vi "MegaAwesome_10_10_12b_JW.vi"() -> ()   [LabVIEW 2011]
uses:
  data/MegaAwesome_States.ctl
  <vilib>/Utility/inputDevices.llb/keyboardAcquire.vi
  <vilib>/Utility/file.llb/Read From Spreadsheet File (string).vi
  <vilib>/Utility/file.llb/Write To Spreadsheet File (string).vi
panel:
  out "Save Next?":bool
  out "Image Center X":i32
  in  "Disable Flag":bool
  out "Index":string
  in  "Slider Min":dbl=5.0
  in  "Slider Max":dbl=5.0
  out "Opj X Axis":string
  out "X Axis Display Type":string
  in  "Index-Sat":dbl=5.0
  in  "Index-Lin":dbl=5.0
  in  "IndexLog-Lin":dbl=5.0
  in  "IndexLog-Sat":dbl=5.0 caption="Num Pts"
  out "Lin Id-Log Used":dbl[](array[numeric])
  out "Lin-Vg Array-Log Used":dbl[](array[numeric])
  in  "New: Comments":string
  out "Save Array":string[][](array[string])
  out "Folder Index":i32 caption="Length"
  out "Sat Id-Used":dbl[](array[numeric])
  out "Sat Vg Array-Used":dbl[](array[numeric])
  out "Vg Array-Log-Used":dbl[](array[numeric])
  out "Sat Id-Log-Used":dbl[](array[numeric])
  out "Lin Id-Used":dbl[](array[numeric])
  out "Lin-Vg Array-Used":dbl[](array[numeric])
  out "Lin Vd":dbl
  out "Recorded Prop":T1
  out "Current State":T2
  in  "Main Tab Control":T3(tab)
  in  "Transfer File":path
  out "Transfer Folder":path
  in  "Transport\nFolder":path caption="Transport Folder"
  out "Transport\nFile":path caption="Transport File"
  in  "Image Folder":path
  out "Image File":path
  out "Fabrication Prop":T4
  out "Distances":i32[](array[numeric])
  in  "Zoom":i32(slide)=-3 scale=-5.0..5.0
  in  "Magnification":i32(ring) items=["5x", "10x", "20x", "50x", "80x"]
  in  "Undo Button":bool
  in  "Remove Button":bool
  in  "Transfer Plots":T5(tab)=enum."Saturation"
  in  "Lin-Trans Slider":dbl(slide) step=1.0 scale=-40.0..40.0 scale format="%#_1p"
  out "Sqrt-Lin":cluster{dbl[], dbl[]}[](graph)
  in  "Sat-Trans Slider":dbl(slide) step=1.0 scale=-40.0..40.0 scale format="%#_1p"
  out "Sqrt-Sat":cluster{dbl[], dbl[]}[](graph)
  out "Raw- Lin":cluster{dbl[], dbl[]}[](graph)
  out "Raw- Sat":cluster{dbl[], dbl[]}[](graph)
  in  "Log Plots":enum32{"Linear", "Saturation", "Transport"}(tab)=enum."Saturation"
  in  "Lin-Log Slider":dbl(slide) step=1.0 scale=-40.0..40.0 scale format="%#_1p"
  out "Lin-Log":cluster{dbl[], dbl[]}[](graph)
  in  "Sat-Log Slider":dbl(slide) step=1.0 scale=-40.0..40.0 scale format="%#_1p"
  out "Sat-Log":cluster{dbl[], dbl[]}[](graph)
  out "Transport":cluster{ext[], ext[]}[](graph)
  out "Transport Name:":string
  in  "Manual Controls":T6
  in  "File Controls":T7
  out "Date Recorded":string="Date Recorded" caption="Measured"
  out "Data Name:":string
  out "Image Name":string
  out "Date Created":string caption="Fabricated"
  in  "Comments:":string
  out "Rec: Length":dbl caption="Length" format="%#_3g"
  out "Rec: Width":dbl caption="Width" format="%#_4g"
  out "Rec: Dielectric (d)":dbl caption="Dielectric (d)" format="%#_3g"
  in  "New: Dielectric":dbl
  in  "New: Length":dbl
  in  "New: Width":dbl
  out "Rec: Temp":dbl caption="Sample Temp" format="%.1f"
  in  "New: Temp":dbl format="%.1f"
  out "Image Out":T8(plugin-control)
  in  "Num Pts":dbl=5.0
  in  "Num Pts Log":dbl=5.0 caption="Num Pts"
  out "Recorded Values Cluster":T9
  out "Calculated Values Cluster":T9 caption="Recorded Values Cluster"
  out "Re-Calculated Values Cluster":T9 caption="Recorded Values Cluster"
  in  "Independant Variable:":string(combo)="Length (um):"
  out "Image Preview":T8(plugin-control)
  out "Total Width":i32
  in  "Index Array":i32(ring) caption="Index" items=["4C", "4C", "4C", "4C", "4C", "4C", "4C", "4C", "4C", "4C", "4C", "4C", "4C", "4C", "4C", "4C", "4C", "4C", "4C", "4C", "4C", "4C", "4C", "4C", "4C", "4C", "4C", "4C", "4C", "4C", "4C", "4C", "4C", "4C", "4C", "4C", "4C", "4C", "4C"]
  in  "Room Temp":dbl=294.0 caption="Room Temp (K)"
  out "No Image\n File":path=path "\\\\acad1\\physics/Jurchescu-group/JW-PD/Mega Awesome/Image Not Found.png" caption="No Image File"
  out "Origin Project File":path=path "\\\\acad1\\physics/Jurchescu-group/JW-PD/Group Library/Origin Project Files/DeviceData_8_10_12a_JW.opj"
  out "No Transport\n File":path=path "\\\\acad1\\physics/Jurchescu-group/JW-PD/Mega Awesome/No Transport File.txt" caption="No Transport File"
  in  "Transport Style Controls":T10={"Transport Line Size"=1, "Transport Line Color"=16772608} {"Transport Line Size" items=["Extra Small", "Small", "Medium", "Large", "Extra Large"]}
  out "Application Directory":path
  # "1)  Select the Transfer File that you would like to analyze:"
  # "Transfer Location"
  # "2) What else would you like to view during your analysis?"
  # "Transport Location"
  # "Image Location"
  # "Recorded"
  # "Calculated"
  # "Re-Calculated"
  # "Manual"
  # "um"
  # "Slider\nDoesn't\nWork"
  # "V"
  # "V"
  # "Slider\nDoesn't\nWork"
  # "V"
  # "Default File Choices"
  # "Default Analysis Values"
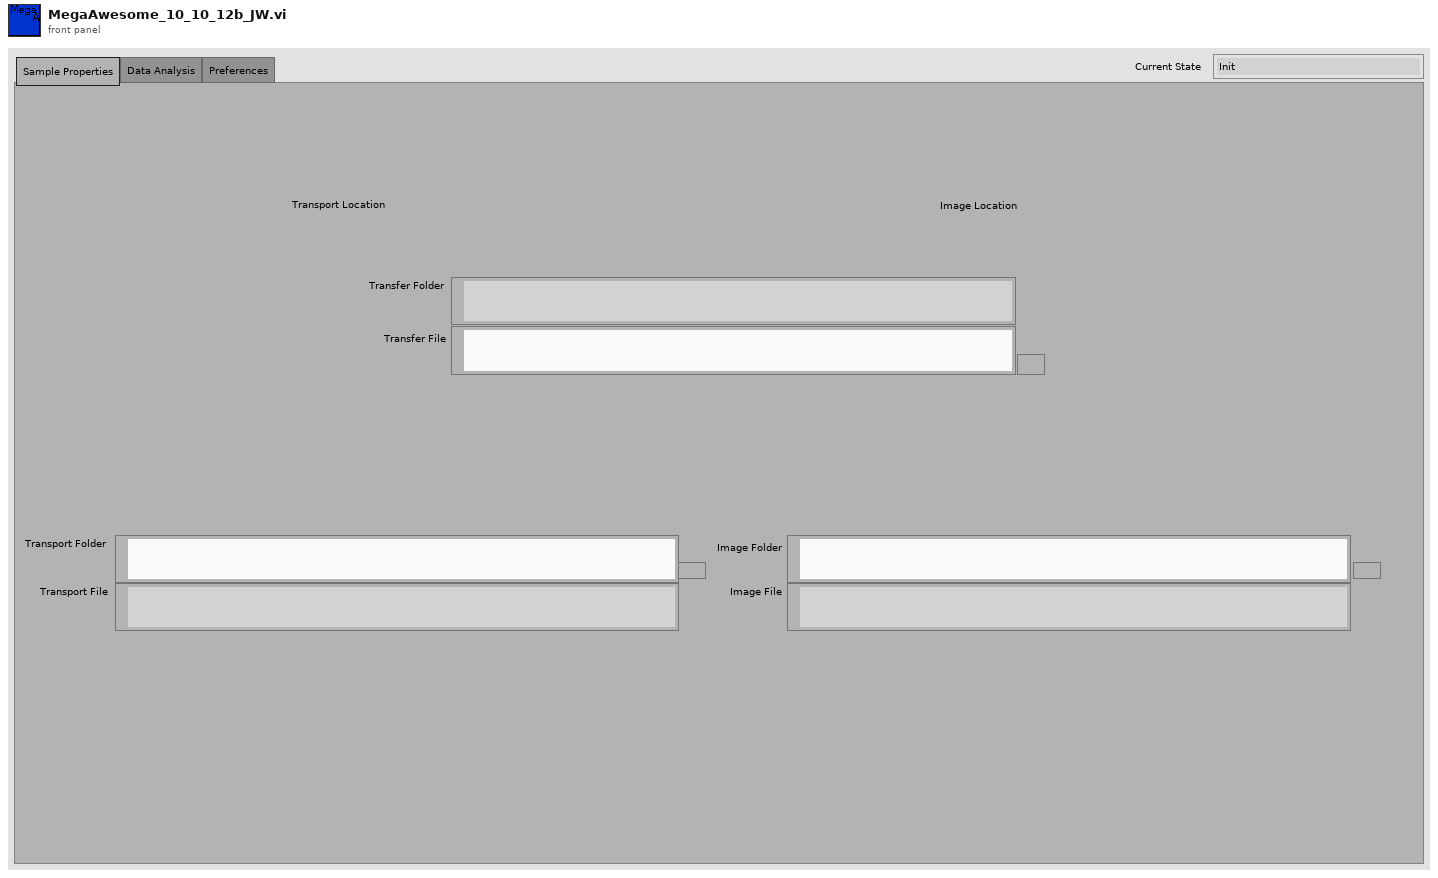
[diagram p1: front panel]
types:
  T1 = cluster{"Date Recorded":string, "Index":string, "Length":dbl, "Width":dbl, "Sample Temp":dbl}
  T2 = typedef "MegaAwesome_States.ctl" = enum16{"Init", "File Missing", "No Event", "Read Data", "Calculated Values", "Re-Calculated Values", "Next File", "Previous File", "Discard File", "Save", "Save Lines", "Export", "Exit"}
  T3 = enum32{"Sample Properties", "Data Analysis", "Preferences"}
  T4 = cluster{"Date Created":string, "Material":string, "Solvent":string, "Concentration":dbl, "Method":string, "Dielectric (nm)":dbl, "Treatment":string, "Comments":string}
  T5 = enum32{"Linear", "Saturation", "Raw-Linear", "Raw-Saturation"}
  T6 = cluster{"Manual-Temp":bool, "Manual-Width":bool, "Manuel-Length":bool, "Manuel-Dielectric":bool, "Manual Comments":bool}
  T7 = cluster{"Previous File":bool, "Discard ":bool, "Save Lines":bool, "Close":bool, "Next File ":bool, "Save":bool, "Save Next":bool, "Export":bool}
  T8 = typedef "IMAQ Image.ctl" = refnum<image>
  T9 = cluster{"Mobility-Sat":dbl, "Moblitity-Lin":dbl, "On/Off":dbl, "Off Current":dbl, "Vt-Sat":dbl, "STS":dbl, "Trap Density-VT":dbl, "Trap Density-STS":dbl}
  T10 = cluster{"Transport Line Size":u16, "Transport Line Color":u32}
  T11 = typedef "LVBoundsTypeDef.ctl" = cluster{"Width":u32, "Height":u32}
  T12 = enum16{"0", "1", "2", "3", "4", "5", "6", "7", "8", "9", "A", "B", "C", "D", "E", "F", "G", "H", "I", "J", "K", "L", "M", "N", "O", "P", "Q", "R", "S", "T", "U", "V", "W", "X", "Y", "Z", "F1", "F2", "F3", "F4", "F5", "F6", "F7", "F8", "F9", "F10", "F11", "F12", "F13", "F14", "F15", "ADD", "BACK", "BACKSLASH", "CAPITAL", "COMMA", "DECIMAL", "DELETE", "DIVIDE", "DOWN", "END", "EQUALS", "ESCAPE", "GRAVE (`)", "HOME", "INSERT", "LBRACKET", "LCONTROL", "LEFT", "L ALT", "LSHIFT", "LWIN", "MINUS", "MULTIPLY", "NEXT", "NUMLOCK", "NUMPAD_0", "NUMPAD_1", "NUMPAD_2", "NUMPAD_3", "NUMPAD_4", "NUMPAD_5", "NUMPAD_6", "NUMPAD_7", "NUMPAD_8", "NUMPAD_9", "PAUSE", "PERIOD", "PRIOR (PG UP)", "RBRACKET", "RCONTROL", "RETURN", "RIGHT", "R ALT", "RSHIFT", "RWIN", "SCROLL", "SEMICOLON", "SLASH", "SPACE", "SUBTRACT", "TAB", "UP", "ENTER (num pad)", "' (quote)"}[]
  T13 = enum16{"0", "1", "2", "3", "4", "5", "6", "7", "8", "9", "A", "B", "C", "D", "E", "F", "G", "H", "I", "J", "K", "L", "M", "N", "O", "P", "Q", "R", "S", "T", "U", "V", "W", "X", "Y", "Z", "F1", "F2", "F3", "F4", "F5", "F6", "F7", "F8", "F9", "F10", "F11", "F12", "F13", "F14", "F15", "ADD", "BACK", "BACKSLASH", "CAPITAL", "COMMA", "DECIMAL", "DELETE", "DIVIDE", "DOWN", "END", "EQUALS", "ESCAPE", "GRAVE (`)", "HOME", "INSERT", "LBRACKET", "LCONTROL", "LEFT", "L ALT", "LSHIFT", "LWIN", "MINUS", "MULTIPLY", "NEXT", "NUMLOCK", "NUMPAD_0", "NUMPAD_1", "NUMPAD_2", "NUMPAD_3", "NUMPAD_4", "NUMPAD_5", "NUMPAD_6", "NUMPAD_7", "NUMPAD_8", "NUMPAD_9", "PAUSE", "PERIOD", "PRIOR (PG UP)", "RBRACKET", "RCONTROL", "RETURN", "RIGHT", "R ALT", "RSHIFT", "RWIN", "SCROLL", "SEMICOLON", "SLASH", "SPACE", "SUBTRACT", "TAB", "UP", "ENTER (num pad)", "' (quote)"}
  T14 = typedef "ROI Descriptor" = cluster{"Global Rectangle":i32[], "Contours":cluster{"ID":enum32{"External", "Internal"}, "Type":u32, "Coordinates":i32[]}[]}
  T15 = cluster{string, dbl, bool, bool, bool, bool, bool, bool, i32}
  T16 = cluster{i32, cluster{string, dbl, bool, bool, bool, bool, bool, bool, i32}, i32, i32}
  T17 = cluster{"Global Rectangle":i32[], "Contours":cluster{"Contour Type":u32, "ROI Type":u32, "Points":i32[]}[]}
  T18 = cluster{"Contour Type":u32, "ROI Type":u32, "Points":i32[]}[]
  T19 = cluster{"[0]":cluster{dbl[], dbl[]}, "[1]":cluster{dbl[], dbl[]}, "[2]":cluster{dbl[], dbl[]}, "[3]":cluster{dbl[], dbl[]}, "[4]":cluster{dbl[], dbl[]}, "[5]":cluster{dbl[], dbl[]}, "[6]":cluster{dbl[], dbl[]}, "[7]":cluster{dbl[], dbl[]}, "[8]":cluster{dbl[], dbl[]}}
  T20 = cluster{i32[], cluster{"Contour Type":u32, "ROI Type":u32, "Points":i32[]}[]}
  T21 = cluster{"Contour Type":u32, "ROI Type":u32, "Points":i32[]}
  T22 = cluster{"Points[0]":i32, "Points[1]":i32, "Points[2]":i32, "Points[3]":i32, "Points[4]":i32, "Points[5]":i32, "Points[6]":i32, "Points[7]":i32, "Points[8]":i32}
  T23 = cluster{"Sat Vg Used":dbl[], "Sat Sqrt(Id) Used ":dbl[], "Lin Vg Used":dbl[], "Lin Sqrt(Id) Used":dbl[], "Index-Lin":dbl, "Index-Sat":dbl}
  T24 = cluster{"Raw Sat":cluster{dbl[], dbl[]}[], "Sqrt Sat":cluster{dbl[], dbl[]}[], "Log Sat":cluster{dbl[], dbl[]}[], "Raw Lin":cluster{dbl[], dbl[]}[], "Sqrt Lin":cluster{dbl[], dbl[]}[], "Log Lin":cluster{dbl[], dbl[]}[]}
  T25 = cluster{"Mobility-Sat":dbl, "Vt-Sat":dbl, "Mobility-Lin":dbl, "Vt-Lin":dbl, "Off I-Sat":dbl, "On/Off I-Sat":dbl}
  T26 = cluster{"Sat Vg Used":dbl[], "Sat Log(Id) Used":dbl[], "Lin Vg Used":dbl[], "Lin Log(Id) Used":dbl[], "STS Index-Sat":dbl, "STS Index-Lin":dbl}
  T27 = cluster{"Independant  Variable Indicator":string, "Parameter String Indicator":string}
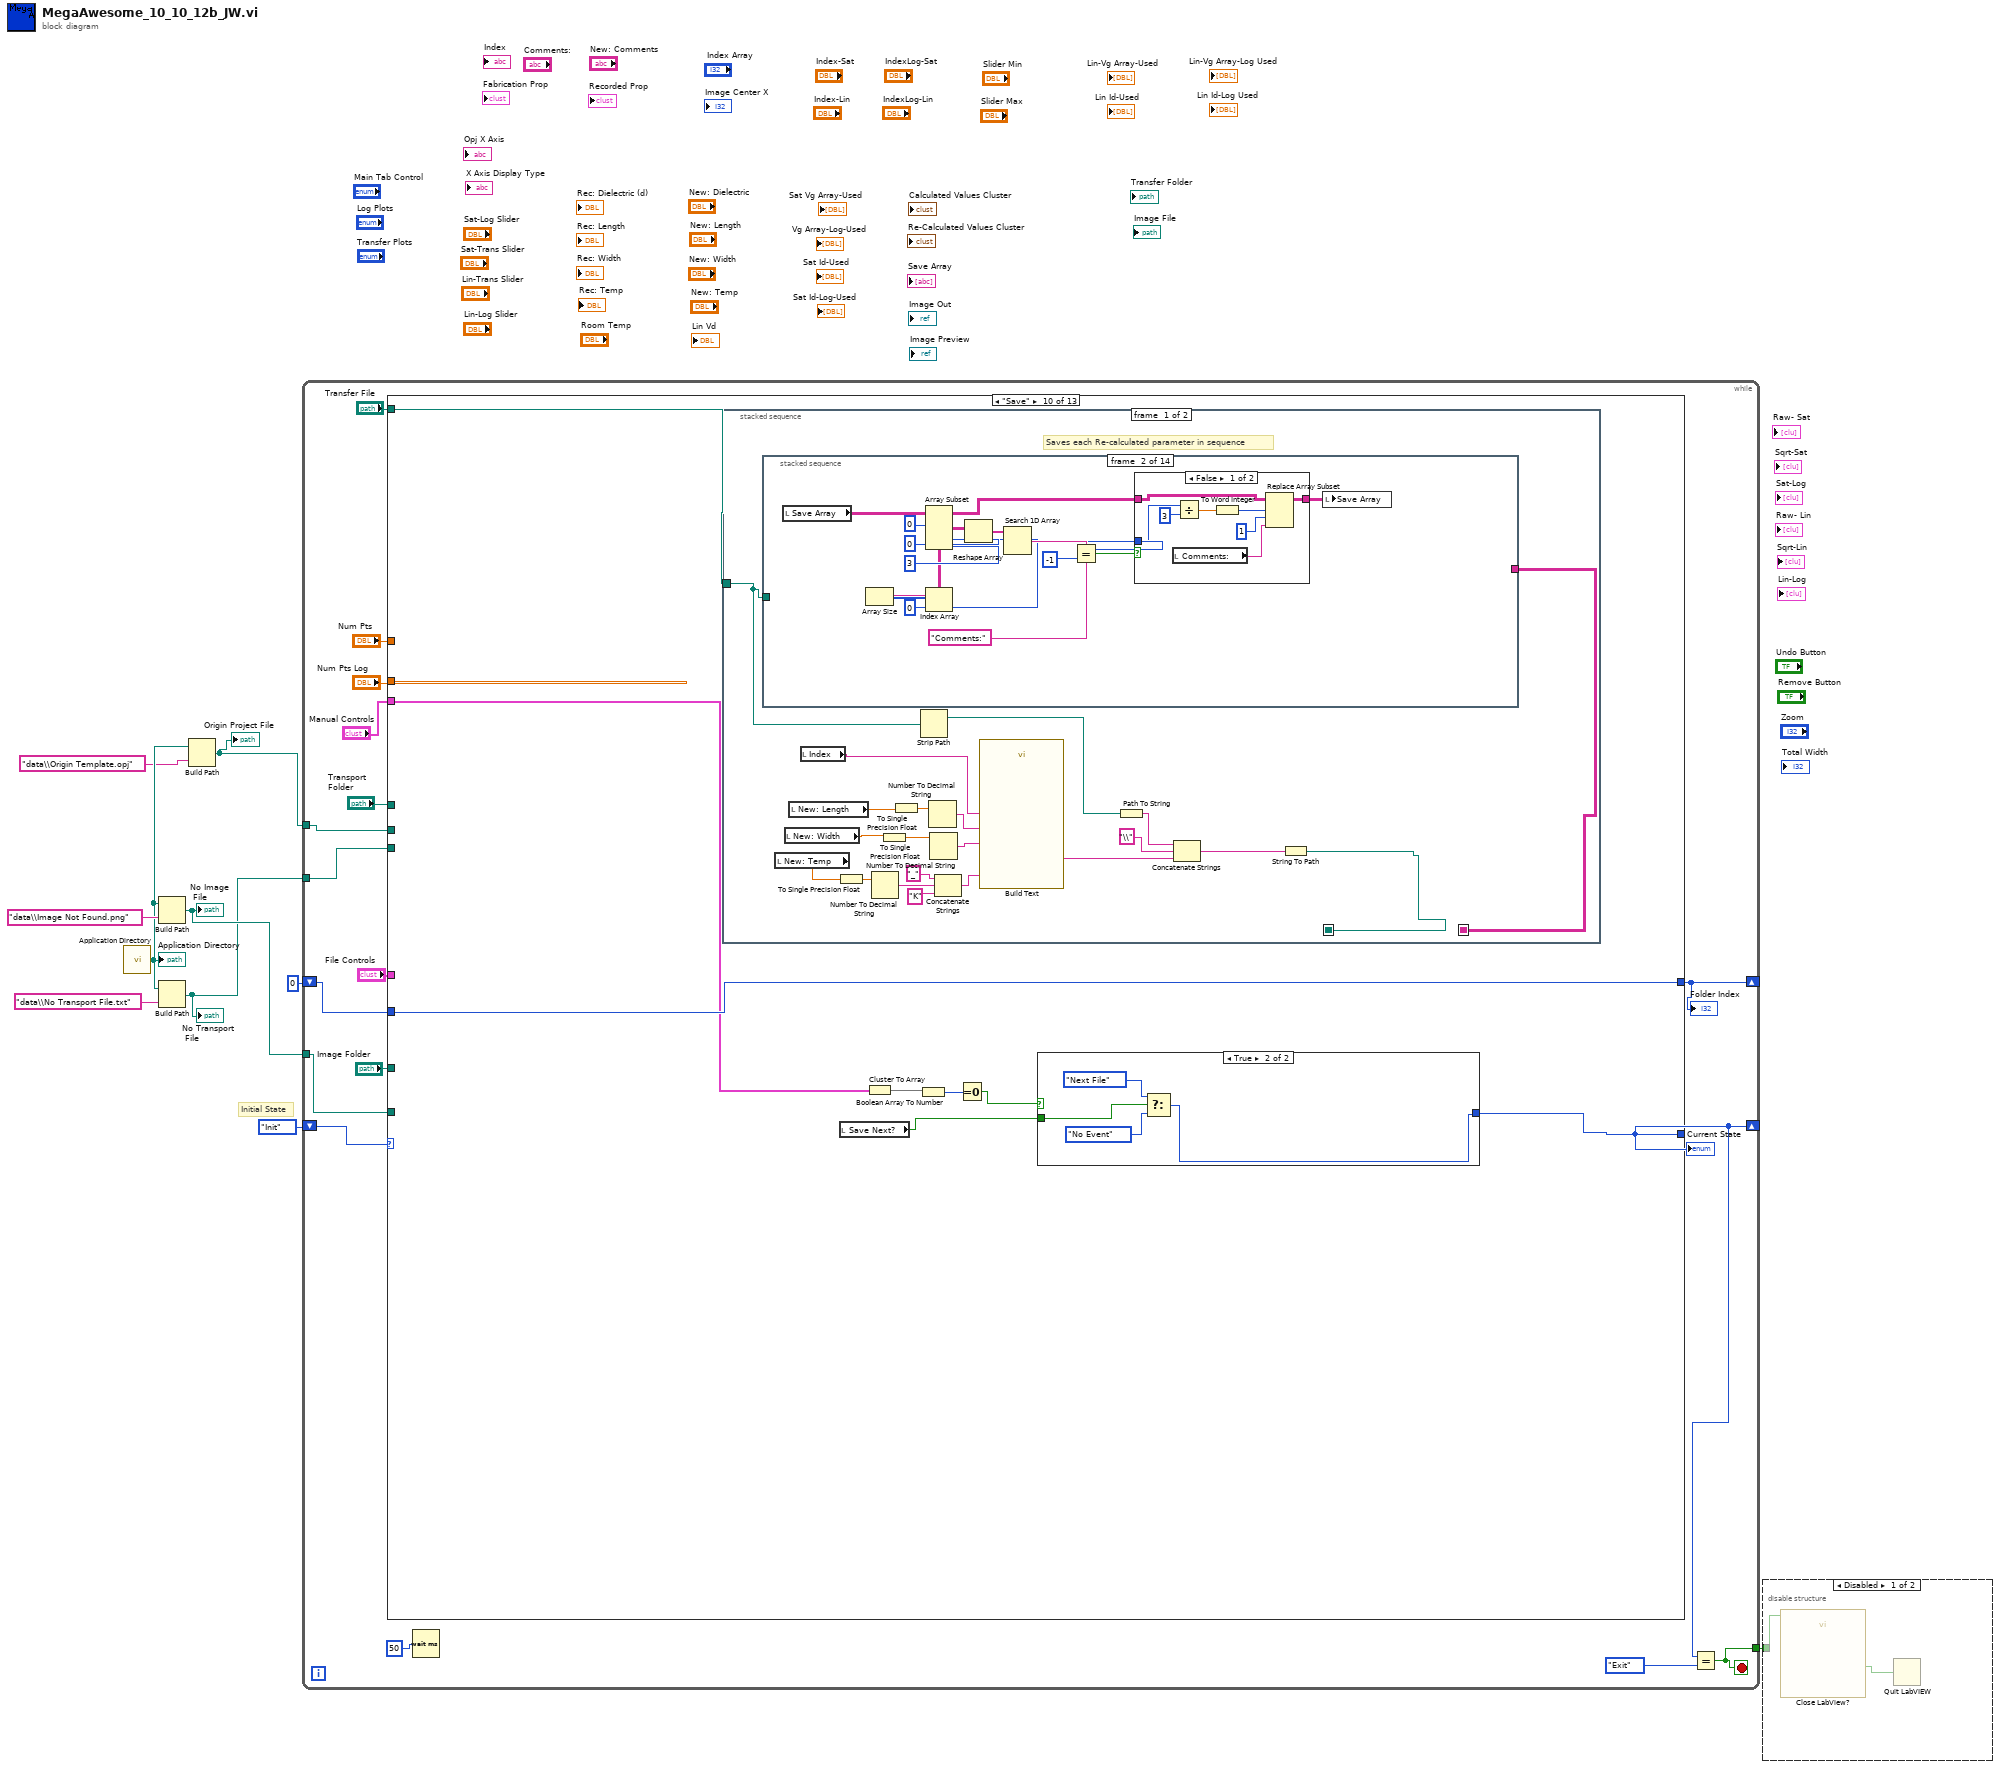
[diagram p0: block diagram]
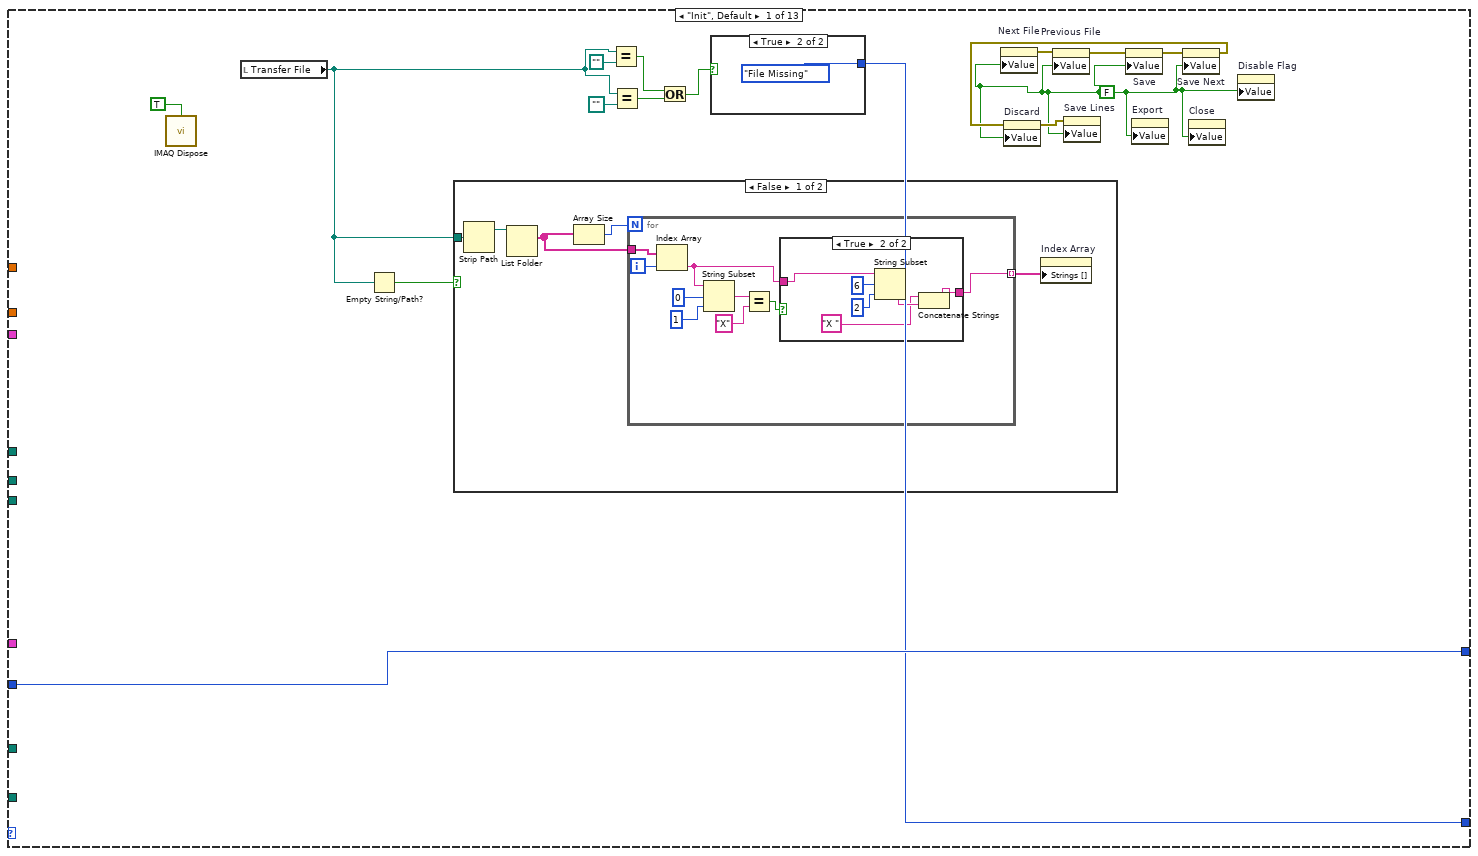
[diagram p3: hidden frame]
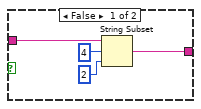
[diagram p4: hidden frame]
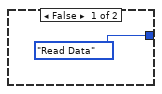
[diagram p6: hidden frame]
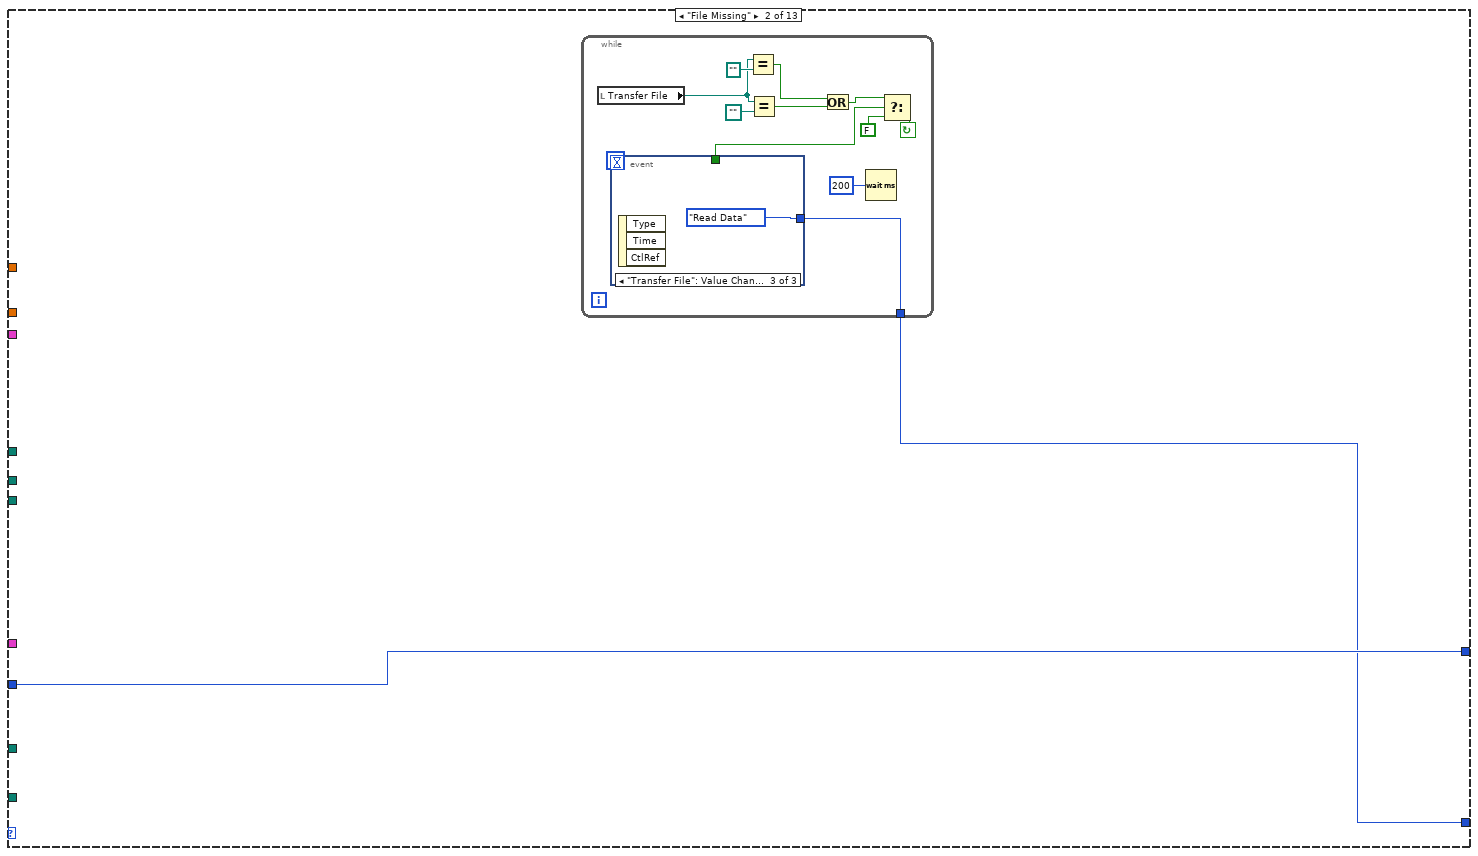
[diagram p7: hidden frame]
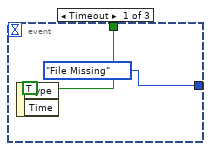
[diagram p8: hidden frame]
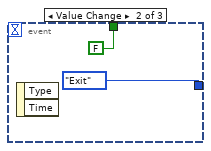
[diagram p9: hidden frame]
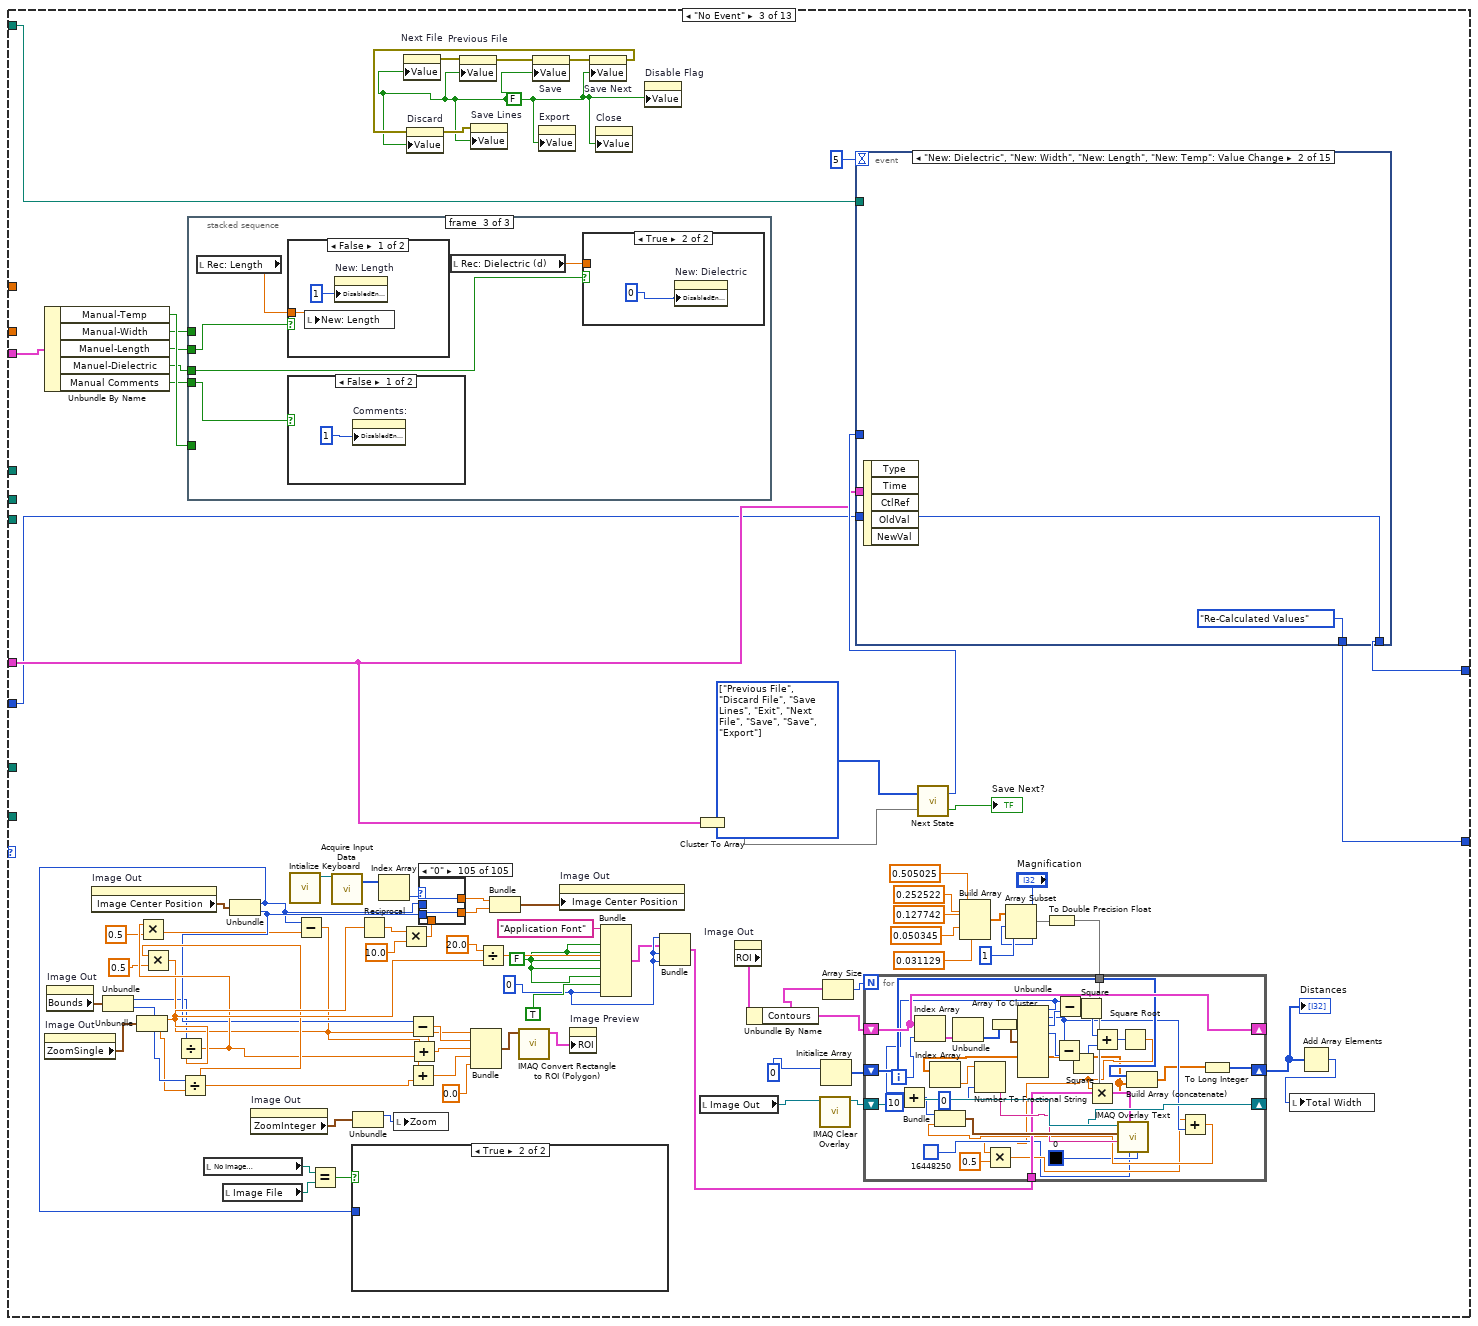
[diagram p10: hidden frame]
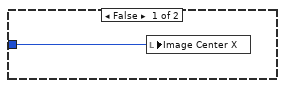
[diagram p11: hidden frame]
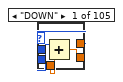
[diagram p12: hidden frame]
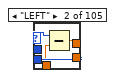
[diagram p13: hidden frame]
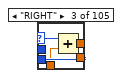
[diagram p14: hidden frame]
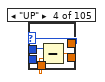
[diagram p15: hidden frame]
diagram:
  # "Initial State"
  n1 = call <vilib>:"Application Directory.vi"() -> ("Application Directory"=w3:path)
  "Application Directory" <- w3
  n2 = Build Path(base path=w3, name or relative path="data\\Image Not Found.png") -> (appended path=w6:path)
  "No Image\n File" <- w6
  n3 = Build Path(base path=w3, name or relative path="data\\No Transport File.txt") -> (appended path=w5:path)
  "No Transport\n File" <- w5
  n4 = Build Path(base path=w3, name or relative path="data\\Origin Template.opj") -> (appended path=w4:path)
  "Origin Project File" <- w4
  n5 = while {
    shift-right: [w11] -> _
    shift-left: MegaAwesome_States."Init" -> [w13]
    shift-right: [w21] -> _
    shift-left: 0 -> [w22]
    tunnel: w6 -> [w18]
    tunnel: w5 -> [w16]
    tunnel: w4 -> [w15]
    tunnel: [w14] -> w1
    stop <- w14 stop-if-true
    n6 = case shown="\"Save\"" w13 {
      tunnel: [w28 w70 w164 MegaAwesome_States."Calculated Values" MegaAwesome_States."Re-Calculated Values" MegaAwesome_States."No Event" MegaAwesome_States."Read Data" MegaAwesome_States."Read Data" MegaAwesome_States."Init" w816 MegaAwesome_States."Exit" MegaAwesome_States."No Event" MegaAwesome_States."No Event"] -> w11
      tunnel: "Transfer File" -> [_ _ w156 w615 w663 _ w764 w775 w802 w821 _ _ _]
      tunnel: "Num Pts" -> [_ _ _ _ w698 _ _ _ _ _ _ _ _]
      tunnel: "Num Pts Log" -> [_ _ _ _ w697 _ _ _ _ _ _ _ _]
      tunnel: "Image Folder" -> [_ _ _ _ w694 _ _ _ _ _ _ w1351 _]
      tunnel: w18 -> [_ _ _ _ w693 _ _ _ _ _ _ _ _]
      tunnel: [w38 w71 w157 w620 w692 w724 w750 w773 w798 w822 w1337 w1361 w1367] -> w21
      tunnel: w22 -> [w38 w71 w89 w618 w692 w724 w751 w774 _ w822 w1337 w1361 w1367]
      tunnel: "Manual Controls" -> [_ _ w166 _ _ _ _ _ _ w820 _ _ _]
      tunnel: "File Controls" -> [_ _ w154 _ _ _ _ _ _ _ _ _ _]
      tunnel: "Transport\nFolder" -> [_ _ _ _ w659 _ _ _ _ _ _ _ _]
      tunnel: w16 -> [_ _ _ _ w658 _ _ _ _ _ _ _ _]
      tunnel: w15 -> [_ _ _ _ _ _ _ _ _ _ _ _ w1366]
      frame "Init", Default {
        w29 = FALSE
        n7 = call "IMAQ Dispose"("All Images? (No)"=TRUE) -> ()  [unwired: 5 in, 1 out]
        n8 = local read "Transfer File"() -> (w36:path)
        n9 = Empty String/Path?(string/path=w36) -> (empty?=w37:bool)
        n10 = case shown="False" w37 {
          tunnel: w36 -> [w45 _]
          frame False {
            n11 = Strip Path(path=w45) -> (stripped path=w47:path)  [unwired: 1 out]
            n12 = List Folder(path=w47) -> (filenames=w46:string[])  [unwired: 3 in, 3 out]
            n13 = Array Size(array=w46) -> (size(s)=w48:i32)
            n14 = for {
              N: w48 -> [_]
              tunnel: w46 -> [w57]
              tunnel: [w55] -> w44 mode=indexing
              i -> [w56]
              n15 = Index Array(array=w57, index=w56) -> (element=w54:string)
              n16 = String Subset(string=w54, offset (0)=0, length (rest)=1) -> (substring=w51:string)
              n17 = Equal?(x=w51, y="X") -> (x = y?=w50:bool)
              n18 = case shown="True" w50 {
                tunnel: w54 -> [w61 w65]
                tunnel: [w58 w64] -> w55
                frame False {
                  n19 = String Subset(string=w61, offset (0)=4, length (rest)=2) -> (substring=w58:string)
                }
                frame True {
                  n20 = String Subset(string=w65, offset (0)=6, length (rest)=2) -> (substring=w63:string)
                  n21 = Concatenate Strings("X ", w63) -> (w64:string)
                }
              }
            }
            n22 = property on="Index Array" class="Ring (strict)"("Strings []"=w44) -> ()  [unwired: 2 in, 2 out]
          }
          frame True {
          }
        }
        n23 = Equal?(x=w36, y=path "") -> (x = y?=w41:bool)
        n24 = Equal?(x=w36, y=path "") -> (x = y?=w40:bool)
        n25 = Or(x=w41, y=w40) -> (x .or. y?=w43:bool)
        n26 = case shown="True" w43 {
          tunnel: [MegaAwesome_States."Read Data" MegaAwesome_States."File Missing"] -> w28
          frame False {
          }
          frame True {
          }
        }
        n27 = property on="Next File" class="Bool (strict)"("Value"=w29) -> (error out=w34:errorcluster)  [unwired: 2 in, 1 out]
        n28 = property on="Previous File" class="Bool (strict)"(error in=w34, "Value"=w29) -> (error out=w33:errorcluster)  [unwired: 1 in, 1 out]
        n29 = property on="Save" class="Bool (strict)"(error in=w33, "Value"=w29) -> (error out=w32:errorcluster)  [unwired: 1 in, 1 out]
        n30 = property on="Export" class="Bool (strict)"("Value"=w29) -> ()  [unwired: 2 in, 2 out]
        n31 = property on="Save Next" class="Bool (strict)"(error in=w32, "Value"=w29) -> (error out=w31:errorcluster)  [unwired: 1 in, 1 out]
        n32 = property on="Discard" class="Bool (strict)"(error in=w31, "Value"=w29) -> (error out=w30:errorcluster)  [unwired: 1 in, 1 out]
        n33 = property on="Save Lines" class="Bool (strict)"(error in=w30, "Value"=w29) -> ()  [unwired: 1 in, 2 out]
        n34 = property on="Close" class="Bool (strict)"("Value"=w29) -> ()  [unwired: 2 in, 2 out]
        n35 = property on="Disable Flag" class="Bool (strict)"("Value"=w29) -> ()  [unwired: 2 in, 2 out]
      }
      frame "File Missing" {
        n36 = while {
          tunnel: [w78] -> w70
          stop <- w74 continue-if-true
          n37 = local read "Transfer File"() -> (w79:path)
          n38 = event shown="[2] \"Transfer File\": Value Change" {
            selector: _ -> [_ _ _]
            dyn-events: _ -> [_ _ _]
            timeout: 10 -> [_ _ _]
            tunnel: [MegaAwesome_States."File Missing" MegaAwesome_States."Exit" MegaAwesome_States."Read Data"] -> w78
            tunnel: [TRUE FALSE _] -> w77
            event Timeout {
              n39 = event-data() -> ()  [unwired: 1 in, 2 out]
            }
            event "File Controls.Close": Value Change {
              n40 = event-data() -> ()  [unwired: 1 in, 2 out]
            }
            event "Transfer File": Value Change {
              n41 = event-data() -> ()  [unwired: 1 in, 3 out]
            }
          }
          n42 = Equal?(x=w79, y=path "") -> (x = y?=w81:bool)
          n43 = Equal?(x=w79, y=path "") -> (x = y?=w82:bool)
          n44 = Or(x=w81, y=w82) -> (x .or. y?=w76:bool)
          n45 = Wait (ms)(milliseconds to wait=u32 200) -> ()  [unwired: 1 out]
          n46 = Select(t=w76, s=w77, f=FALSE) -> (s? t:f=w74:bool)
        }
      }
      frame "No Event" {
        w145 = FALSE
        w147 = 0
        w155 = FALSE
        w173 = T2[] [enum."Previous File", enum."Discard File", enum."Save Lines", enum."Exit", enum."Next File", enum."Save", enum."Save", enum."Export"] items=["Init", "File Missing", "No Event", "Read Data", "Calculated Values", "Re-Calculated Values", "Next File", "Previous File", "Discard File", "Save", "Save Lines", "Export", "Exit"]
        n47 = Unbundle By Name(w166) -> ("Manual-Temp"=w171:bool, "Manual-Width"=w170:bool, "Manuel-Length"=w169:bool, "Manuel-Dielectric"=w168:bool, "Manual Comments"=w167:bool)
        n48 = property on="Image Out" class="ImageControl"() -> ("ZoomSingle"=w131:cluster{"X":sgl, "Y":sgl})  [unwired: 2 in, 2 out]
        n49 = property on="Image Out" class="ImageControl"() -> ("Bounds"=w130:T11)  [unwired: 2 in, 2 out]
        n50 = property on="Image Out" class="ImageControl"() -> ("Image Center Position"=w124:cluster{"X":u32, "Y":u32})  [unwired: 2 in, 2 out]
        n51 = Unbundle(w130) -> ("Width"=w133:u32, "Height"=w134:u32)
        n52 = Unbundle(w131) -> ("X"=w151:sgl, "Y"=w132:sgl)
        n53 = Divide(x=w133, y=w151) -> (x/y=w142:sgl)
        n54 = Multiply(x=w142, y=0.5) -> (x*y=w137:dbl)
        n55 = Divide(x=w134, y=w132) -> (x/y=w143:sgl)
        n56 = Multiply(x=w143, y=0.5) -> (x*y=w138:dbl)
        n57 = stacked-sequence {
          tunnel: w171 -> [w573 _ _]
          tunnel: w170 -> [_ w587 _]
          tunnel: w169 -> [_ _ w600]
          tunnel: w168 -> [_ _ w598]
          tunnel: w167 -> [_ _ w597]
          frame #0 {
            n58 = local read "Rec: Temp"() -> (w572:dbl)
            n59 = case shown="False" w573 {
              tunnel: w572 -> [w578 _]
              frame False {
                n60 = local read "Rec: Temp"() -> (w576:dbl)
                n61 = property on="New: Temp" class="DigNum (strict)"("DisabledEnum"=1) -> ()  [unwired: 2 in, 2 out]
                n62 = Equal To 0?(x=w576) -> (x = 0?=w577:bool)
                n63 = local write "New: Temp"(w578) -> ()
                n64 = case shown="True" w577 {
                  tunnel: [w579 w580] -> w574
                  tunnel: w576 -> [w579 _]
                  frame False {
                  }
                  frame True {
                    n65 = local read "Room Temp"() -> (w580:dbl)
                  }
                }
                n66 = local write "Rec: Temp"(w574) -> ()
                n67 = local write "New: Temp"(w574) -> ()
              }
              frame True {
                n68 = property on="New: Temp" class="DigNum (strict)"("DisabledEnum"=0) -> ()  [unwired: 2 in, 2 out]
              }
            }
          }
          frame #1 {
            n69 = local read "New: Width"() -> (w588:dbl)
            n70 = local read "Total Width"() -> (w584:i32)
            n71 = case shown="True" w587 {
              frame False {
                n72 = property on="New: Width" class="DigNum (strict)"("DisabledEnum"=1) -> ()  [unwired: 2 in, 2 out]
              }
              frame True {
                n73 = property on="New: Width" class="DigNum (strict)"("DisabledEnum"=0) -> ()  [unwired: 2 in, 2 out]
              }
            }
            n74 = Not(x=w587) -> (.not. x?=w582:bool)
            n75 = Not Equal?(x=w584, y=w588) -> (x != y?=w583:bool)
            n76 = Equal To 0?(x=w584) -> (x = 0?=w586:bool)
            n77 = And(x=w582, y=w586) -> (x .and. y?=w585:bool)
            n78 = case shown="False" w585 {
              tunnel: w584 -> [w592 _]
              tunnel: w583 -> [w591 _]
              tunnel: w582 -> [w590 _]
              frame False {
                n79 = And(x=w590, y=w591) -> (x .and. y?=w589:bool)
                n80 = case shown="True" w589 {
                  tunnel: w592 -> [_ w593]
                  frame False {
                  }
                  frame True {
                    n81 = property on="New: Width" class="DigNum (strict)"("Val(Sgnl)"=w593) -> ()  [unwired: 2 in, 2 out]
                  }
                }
              }
              frame True {
                n82 = local read "Rec: Width"() -> (w594:dbl)
                n83 = local write "New: Width"(w594) -> ()
              }
            }
          }
          frame #2 {
            n84 = local read "Rec: Length"() -> (w601:dbl)
            n85 = case shown="False" w600 {
              tunnel: w601 -> [w608 _]
              frame False {
                n86 = local write "New: Length"(w608) -> ()
                n87 = property on="New: Length" class="DigNum (strict)"("DisabledEnum"=u8 1) -> ()  [unwired: 2 in, 2 out]
              }
              frame True {
                n88 = property on="New: Length" class="DigNum (strict)"("DisabledEnum"=0) -> ()  [unwired: 2 in, 2 out]
              }
            }
            n89 = case shown="False" w597 {
              frame False {
                n90 = property on="Comments:" class="Str"("DisabledEnum"=1) -> ()  [unwired: 2 in, 2 out]
              }
              frame True {
                n91 = property on="Comments:" class="Str"("DisabledEnum"=0) -> ()  [unwired: 2 in, 2 out]
              }
            }
            n92 = local read "Rec: Dielectric (d)"() -> (w599:dbl)
            n93 = case shown="True" w598 {
              tunnel: w599 -> [w605 _]
              frame False {
                n94 = local write "New: Dielectric"(w605) -> ()
                n95 = property on="New: Dielectric" class="DigNum (strict)"("DisabledEnum"=1) -> ()  [unwired: 2 in, 2 out]
              }
              frame True {
                n96 = property on="New: Dielectric" class="DigNum (strict)"("DisabledEnum"=0) -> ()  [unwired: 2 in, 2 out]
              }
            }
          }
        }
        n97 = local read "No Image\n File"() -> (w95:path)
        n98 = local read "Image File"() -> (w94:path)
        n99 = Unbundle(w124) -> ("X"=w96:u32, "Y"=w141:u32)
        n100 = property on="Image Out" class="ImageControl"() -> ("ZoomInteger"=w99:cluster{"X":i32, "Y":i32})  [unwired: 2 in, 2 out]
        n101 = call <vilib>:"Intialize Keyboard.vi"() -> ("device ID"=w121:refnum<k1>)  [unwired: 10 in, 1 out]
        n102 = Subtract(x=w96, y=w137) -> (x-y=w139:dbl)
        n103 = Equal?(x=w95, y=w94) -> (x = y?=w93:bool)
        n104 = call-poly <vilib>:"Acquire Input Data.vi"("device ID"=w121) -> ("keys pressed"=w122:T12)  [unwired: 16 in, 2 out]
        n105 = case shown="True" w93 {
          tunnel: w96 -> [w174 _]
          frame False {
            n106 = local write "Image Center X"(w174) -> ()
          }
          frame True {
          }
        }
        n107 = Unbundle(w99) -> ("X"=w98:i32)  [unwired: 1 out]
        n108 = Reciprocal(x=w151) -> (1/x=w152:sgl)
        n109 = Index Array(array=w122) -> (element=w118:T13)  [unwired: 1 in]
        n110 = local write "Zoom"(w98) -> ()
        n111 = Multiply(x=w152, y=sgl 10.0) -> (x*y=w150:sgl)
        n112 = property on="Next File" class="Bool (strict)"("Value"=w155) -> (error out=w162:errorcluster)  [unwired: 2 in, 1 out]
        n113 = Subtract(x=w141, y=w138) -> (x-y=w140:dbl)
        n114 = Add(x=w140, y=w143) -> (x+y=w126:dbl)
        n115 = Add(x=w139, y=w142) -> (x+y=w125:dbl)
        n116 = case shown="\"0\"" w118 {
          tunnel: w96 -> [w210 w216 w220 w222 w226 w228 w230 w232 w234 w236 w238 w240 w242 w244 w246 w248 w250 w252 w254 w256 w258 w260 w262 w264 w266 w268 w270 w272 w274 w276 w278 w280 w282 w284 w286 w288 w290 w292 w294 w296 w298 w300 w302 w304 w306 w308 w310 w312 w314 w316 w318 w320 w322 w324 w326 w328 w330 w332 w334 w336 w338 w340 w342 w344 w346 w348 w350 w352 w354 w356 w358 w360 w362 w364 w366 w368 w370 w372 w374 w376 w378 w380 w382 w384 w386 w388 w390 w392 w394 w396 w398 w400 w402 w404 w406 w408 w410 w412 w414 w416 w418 w420 w422 w424 w426]
          tunnel: [w210 w215 w219 w222 w226 w228 w230 w232 w234 w236 w238 w240 w242 w244 w246 w248 w250 w252 w254 w256 w258 w260 w262 w264 w266 w268 w270 w272 w274 w276 w278 w280 w282 w284 w286 w288 w290 w292 w294 w296 w298 w300 w302 w304 w306 w308 w310 w312 w314 w316 w318 w320 w322 w324 w326 w328 w330 w332 w334 w336 w338 w340 w342 w344 w346 w348 w350 w352 w354 w356 w358 w360 w362 w364 w366 w368 w370 w372 w374 w376 w378 w380 w382 w384 w386 w388 w390 w392 w394 w396 w398 w400 w402 w404 w406 w408 w410 w412 w414 w416 w418 w420 w422 w424 w426] -> w119
          tunnel: w141 -> [w212 w214 w218 w224 w225 w227 w229 w231 w233 w235 w237 w239 w241 w243 w245 w247 w249 w251 w253 w255 w257 w259 w261 w263 w265 w267 w269 w271 w273 w275 w277 w279 w281 w283 w285 w287 w289 w291 w293 w295 w297 w299 w301 w303 w305 w307 w309 w311 w313 w315 w317 w319 w321 w323 w325 w327 w329 w331 w333 w335 w337 w339 w341 w343 w345 w347 w349 w351 w353 w355 w357 w359 w361 w363 w365 w367 w369 w371 w373 w375 w377 w379 w381 w383 w385 w387 w389 w391 w393 w395 w397 w399 w401 w403 w405 w407 w409 w411 w413 w415 w417 w419 w421 w423 w425]
          tunnel: [w211 w214 w218 w223 w225 w227 w229 w231 w233 w235 w237 w239 w241 w243 w245 w247 w249 w251 w253 w255 w257 w259 w261 w263 w265 w267 w269 w271 w273 w275 w277 w279 w281 w283 w285 w287 w289 w291 w293 w295 w297 w299 w301 w303 w305 w307 w309 w311 w313 w315 w317 w319 w321 w323 w325 w327 w329 w331 w333 w335 w337 w339 w341 w343 w345 w347 w349 w351 w353 w355 w357 w359 w361 w363 w365 w367 w369 w371 w373 w375 w377 w379 w381 w383 w385 w387 w389 w391 w393 w395 w397 w399 w401 w403 w405 w407 w409 w411 w413 w415 w417 w419 w421 w423 w425] -> w120
          tunnel: w150 -> [w209 w213 w217 w221 _ _ _ _ _ _ _ _ _ _ _ _ _ _ _ _ _ _ _ _ _ _ _ _ _ _ _ _ _ _ _ _ _ _ _ _ _ _ _ _ _ _ _ _ _ _ _ _ _ _ _ _ _ _ _ _ _ _ _ _ _ _ _ _ _ _ _ _ _ _ _ _ _ _ _ _ _ _ _ _ _ _ _ _ _ _ _ _ _ _ _ _ _ _ _ _ _ _ _ _ _]
          frame "DOWN" {
            n117 = Add(x=w212, y=w209) -> (x+y=w211:sgl)
          }
          frame "LEFT" {
            n118 = Subtract(x=w216, y=w213) -> (x-y=w215:sgl)
          }
          frame "RIGHT" {
            n119 = Add(x=w220, y=w217) -> (x+y=w219:sgl)
          }
          frame "UP" {
            n120 = Subtract(x=w224, y=w221) -> (x-y=w223:sgl)
          }
          frame "ENTER (num pad)" {
          }
          frame "' (quote)" {
          }
          frame "END" {
          }
          frame "EQUALS" {
          }
          frame "ESCAPE" {
          }
          frame "GRAVE (`)" {
          }
          frame "HOME" {
          }
          frame "INSERT" {
          }
          frame "LBRACKET" {
          }
          frame "LCONTROL" {
          }
          frame "L ALT" {
          }
          frame "LSHIFT" {
          }
          frame "LWIN" {
          }
          frame "MINUS" {
          }
          frame "MULTIPLY" {
          }
          frame "NEXT" {
          }
          frame "NUMLOCK" {
          }
          frame "NUMPAD_0" {
          }
          frame "NUMPAD_1" {
          }
          frame "NUMPAD_2" {
          }
          frame "NUMPAD_3" {
          }
          frame "NUMPAD_4" {
          }
          frame "NUMPAD_5" {
          }
          frame "NUMPAD_6" {
          }
          frame "NUMPAD_7" {
          }
          frame "NUMPAD_8" {
          }
          frame "NUMPAD_9" {
          }
          frame "PAUSE" {
          }
          frame "PERIOD" {
          }
          frame "PRIOR (PG UP)" {
          }
          frame "RBRACKET" {
          }
          frame "RCONTROL" {
          }
          frame "RETURN" {
          }
          frame "R ALT" {
          }
          frame "RSHIFT" {
          }
          frame "RWIN" {
          }
          frame "SCROLL" {
          }
          frame "SEMICOLON" {
          }
          frame "SLASH" {
          }
          frame "SPACE" {
          }
          frame "SUBTRACT" {
          }
          frame "TAB" {
          }
          frame "DIVIDE" {
          }
          frame "DELETE" {
          }
          frame "DECIMAL" {
          }
          frame "COMMA" {
          }
          frame "CAPITAL" {
          }
          frame "BACKSLASH" {
          }
          frame "BACK" {
          }
          frame "ADD" {
          }
          frame "F15" {
          }
          frame "F14" {
          }
          frame "F13" {
          }
          frame "F12" {
          }
          frame "F11" {
          }
          frame "F10" {
          }
          frame "F9" {
          }
          frame "F8" {
          }
          frame "F7" {
          }
          frame "F6" {
          }
          frame "F5" {
          }
          frame "F4" {
          }
          frame "F3" {
          }
          frame "F2" {
          }
          frame "F1" {
          }
          frame "Z" {
          }
          frame "Y" {
          }
          frame "X" {
          }
          frame "W" {
          }
          frame "V" {
          }
          frame "U" {
          }
          frame "T" {
          }
          frame "S" {
          }
          frame "R" {
          }
          frame "Q" {
          }
          frame "P" {
          }
          frame "O" {
          }
          frame "N" {
          }
          frame "M" {
          }
          frame "L" {
          }
          frame "K" {
          }
          frame "J" {
          }
          frame "I" {
          }
          frame "H" {
          }
          frame "G" {
          }
          frame "F" {
          }
          frame "E" {
          }
          frame "D" {
          }
          frame "C" {
          }
          frame "B" {
          }
          frame "A" {
          }
          frame "9" {
          }
          frame "8" {
          }
          frame "7" {
          }
          frame "6" {
          }
          frame "5" {
          }
          frame "4" {
          }
          frame "3" {
          }
          frame "2" {
          }
          frame "1" {
          }
          frame "0" {
          }
        }
        n121 = property on="Previous File" class="Bool (strict)"(error in=w162, "Value"=w155) -> (error out=w161:errorcluster)  [unwired: 1 in, 1 out]
        n122 = Bundle(w139, w140, w125, w126, 0.0) -> (w127:cluster{dbl, dbl, dbl, dbl, dbl})  [unwired: 1 in]
        n123 = Divide(x=20.0, y=w151) -> (x/y=w149:dbl)
        n124 = Bundle("X"=w119, "Y"=w120) -> (w123:cluster{"X":sgl, "Y":sgl})  [unwired: 1 in]
        n125 = call "IMAQ Convert Rectangle to ROI (Polygon)"("Rectangle"=w127) -> ("ROI Descriptor"=w129:T14)  [unwired: 7 in, 2 out]
        n126 = property on="Save" class="Bool (strict)"(error in=w161, "Value"=w155) -> (error out=w160:errorcluster)  [unwired: 1 in, 1 out]
        n127 = property on="Export" class="Bool (strict)"("Value"=w155) -> ()  [unwired: 2 in, 2 out]
        n128 = property on="Image Out" class="ImageControl"("Image Center Position"=w123) -> ()  [unwired: 2 in, 2 out]
        n129 = property on="Image Preview" class="ImageControl"("ROI"=w129) -> ()  [unwired: 2 in, 2 out]
        n130 = property on="Save Next" class="Bool (strict)"(error in=w160, "Value"=w155) -> (error out=w159:errorcluster)  [unwired: 1 in, 1 out]
        n131 = property on="Discard" class="Bool (strict)"(error in=w159, "Value"=w155) -> (error out=w158:errorcluster)  [unwired: 1 in, 1 out]
        n132 = property on="Save Lines" class="Bool (strict)"(error in=w158, "Value"=w155) -> ()  [unwired: 1 in, 2 out]
        n133 = property on="Close" class="Bool (strict)"("Value"=w155) -> ()  [unwired: 2 in, 2 out]
        n134 = Bundle("Application Font", w149, w145, w145, w145, w145, w145, TRUE, w147) -> (w144:T15)  [unwired: 1 in]
        n135 = property on="Disable Flag" class="Bool (strict)"("Value"=w155) -> ()  [unwired: 2 in, 2 out]
        n136 = Bundle(w147, w144, w147, w147) -> (w101:T16)  [unwired: 1 in]
        n137 = Cluster To Array(cluster=w154) -> (array=w172:bool[])
        n138 = local read "Image Out"() -> (w100:T8)
        n139 = property on="Image Out" class="ImageControl"() -> ("ROI"=w103:T17)  [unwired: 2 in, 2 out]
        n140 = Unbundle By Name(w103) -> ("Contours"=w104:T18)
        n141 = call "IMAQ Clear Overlay"("Image"=w100) -> ("Image Out"=w117:T8)  [unwired: 9 in, 1 out]
        n142 = Initialize Array(0) -> (w106:i32[])  [unwired: 1 in]
        n143 = Array Size(array=w104) -> (size(s)=w105:i32)
        n144 = call "Next State.vi"("Buttons []"=w172, "States []"=w173) -> ("Save Next?"=→"Save Next?":bool, "Enum"=w165:T2)
        n145 = event shown="[1] \"New: Dielectric\", \"New: Width\", \"New: Length\", \"New: Temp\": Value Change" {
          selector: _ -> [_ _ _ _ _ _ _ _ _ _ _ _ _ _ _]
          dyn-events: _ -> [_ _ _ _ _ _ _ _ _ _ _ _ _ _ _]
          timeout: 5 -> [_ _ _ _ _ _ _ _ _ _ _ _ _ _ _]
          tunnel: w165 -> [w428 _ _ _ _ _ _ _ _ _ _ _ _ _ _]
          tunnel: [w428 MegaAwesome_States."Re-Calculated Values" MegaAwesome_States."Calculated Values" MegaAwesome_States."Re-Calculated Values" MegaAwesome_States."Re-Calculated Values" MegaAwesome_States."Re-Calculated Values" MegaAwesome_States."Re-Calculated Values" MegaAwesome_States."Read Data" MegaAwesome_States."Read Data" MegaAwesome_States."No Event" MegaAwesome_States."No Event" MegaAwesome_States."No Event" MegaAwesome_States."No Event" MegaAwesome_States."No Event" MegaAwesome_States."No Event"] -> w164
          tunnel: w89 -> [w427 w429 w431 w433 w458 w486 w510 _ w538 w540 w553 w555 w559 w563 w567]
          tunnel: [w427 w429 w431 w433 w458 w486 w510 w529 w538 w540 w553 w555 w559 w563 w567] -> w157
          tunnel: w156 -> [_ _ _ _ _ _ _ w528 _ _ _ _ _ _ _]
          tunnel: w154 -> [_ _ _ _ _ _ _ _ _ _ _ _ _ _ _]
          event Timeout {
            n146 = event-data() -> ()  [unwired: 1 in, 2 out]
          }
          event "New: Dielectric", "New: Width", "New: Length", "New: Temp": Value Change {
            n147 = event-data() -> ()  [unwired: 1 in, 5 out]
          }
          event "Num Pts Log", "Transport Style Controls", "Num Pts": Value Change {
            n148 = event-data() -> ()  [unwired: 1 in, 5 out]
          }
          event "Sat-Trans Slider": Value Change {
            n149 = event-data() -> ()  [unwired: 1 in, 5 out]
            n150 = local read "Sqrt-Sat"() -> (w457:cluster{dbl[], dbl[]}[])
            n151 = Decimate 1D Array(w457) -> (w441:cluster{dbl[], dbl[]}[], w442:cluster{dbl[], dbl[]}[])
            n152 = local read "Slider Min"() -> (w438:dbl)
            n153 = local read "Sat-Trans Slider"() -> (w436:dbl)
            n154 = Array To Cluster(array=w441) -> (cluster=w456:T19)
            n155 = local read "New: Dielectric"() -> (w451:dbl)
            n156 = local read "Num Pts"() -> (w434:dbl)
            n157 = local read "New: Width"() -> (w453:dbl)
            n158 = local read "New: Length"() -> (w452:dbl)
            n159 = Unbundle(w456) -> ("[0]"=w455:cluster{dbl[], dbl[]})  [unwired: 8 out]
            n160 = Absolute Value(x=w438) -> (abs(x)=w437:dbl)
            n161 = Unbundle(w455) -> (w439:dbl[], w454:dbl[])
            n162 = Add(x=w436, y=w437) -> (x+y=w435:dbl)
            n163 = Array Subset(array=w439, index=w435, length=w434) -> (w449:dbl[])
            n164 = local write "Sat Vg Array-Used"(w449) -> ()
            n165 = Array Subset(array=w454, index=w435, length=w434) -> (w450:dbl[])
            n166 = call "Mobility-Vt-Used Pts_Saturation.vi"("Width"=w453, "Length"=w452, "Dielectric (d)"=w451, "Sat Id Used"=w450, "Vg Used"=w449) -> ("Vt"=w445:dbl, "Mobility"=w446:dbl)  [unwired: 4 in, 1 out]
            n167 = local write "Index-Sat"(w435) -> ()
            n168 = local write "Sat Id-Used"(w450) -> ()
            n169 = Bundle(w449, w450) -> (w443:cluster{dbl[], dbl[]})  [unwired: 1 in]
            n170 = local read "Re-Calculated Values Cluster"() -> (w448:T9)
            n171 = Bundle By Name(cluster=w448, "Mobility-Sat"=w446, "Vt-Sat"=w445) -> (w447:T9)
            n172 = local write "Re-Calculated Values Cluster"(w447) -> ()
            n173 = Build Array (concatenate)(w441, w442, w443) -> (w440:cluster{dbl[], dbl[]}[])
            n174 = local write "Sqrt-Sat"(w440) -> ()
          }
          event "Lin-Trans Slider": Value Change {
            n175 = event-data() -> ()  [unwired: 1 in, 5 out]
            n176 = local read "Sqrt-Lin"() -> (w482:cluster{dbl[], dbl[]}[])
            n177 = Decimate 1D Array(w482) -> (w467:cluster{dbl[], dbl[]}[], w468:cluster{dbl[], dbl[]}[])
            n178 = local read "Slider Min"() -> (w464:dbl)
            n179 = Array To Cluster(array=w467) -> (cluster=w481:T19)
            n180 = local read "Lin-Trans Slider"() -> (w462:dbl)
            n181 = local read "New: Dielectric"() -> (w475:dbl)
            n182 = local read "Num Pts"() -> (w478:dbl)
            n183 = local read "New: Width"() -> (w477:dbl)
            n184 = local read "New: Length"() -> (w476:dbl)
            n185 = local read "Lin Vd"() -> (w459:dbl)
            n186 = Unbundle(w481) -> ("[0]"=w480:cluster{dbl[], dbl[]})  [unwired: 8 out]
            n187 = Absolute Value(x=w464) -> (abs(x)=w463:dbl)
            n188 = Unbundle(w480) -> (w465:dbl[], w479:dbl[])
            n189 = Add(x=w462, y=w463) -> (x+y=w461:dbl)
            n190 = Array Subset(array=w465, index=w461, length=w478) -> (w473:dbl[])
            n191 = local write "Lin-Vg Array-Used"(w473) -> ()
            n192 = Array Subset(array=w479, index=w461, length=w478) -> (w474:dbl[])
            n193 = call "Mobility-Vt-Used Pts_Linear.vi"("Width"=w477, "Length"=w476, "Vd"=w459, "Dielectric (d)"=w475, "Id Used"=w474, "Vg Used"=w473) -> ("Mobility"=w470:dbl)  [unwired: 3 in, 2 out]
            n194 = local write "Index-Lin"(w461) -> ()
            n195 = local write "Lin Id-Used"(w474) -> ()
            n196 = Bundle(w473, w474) -> (w469:cluster{dbl[], dbl[]})  [unwired: 1 in]
            n197 = local read "Re-Calculated Values Cluster"() -> (w472:T9)
            n198 = Bundle By Name(cluster=w472, "Moblitity-Lin"=w470) -> (w471:T9)
            n199 = local write "Re-Calculated Values Cluster"(w471) -> ()
            n200 = Build Array (concatenate)(w467, w468, w469) -> (w466:cluster{dbl[], dbl[]}[])
            n201 = local write "Sqrt-Lin"(w466) -> ()
          }
          event "Sat-Log Slider": Value Change {
            n202 = event-data() -> ()  [unwired: 1 in, 5 out]
            n203 = local read "Sat-Log"() -> (w489:cluster{dbl[], dbl[]}[])
            n204 = Decimate 1D Array(w489) -> (w496:cluster{dbl[], dbl[]}[], w497:cluster{dbl[], dbl[]}[])
            n205 = local read "Slider Min"() -> (w493:dbl)
            n206 = Array To Cluster(array=w496) -> (cluster=w506:T19)
            n207 = property on="Sat-Log" class="XYGraph (strict)"("Active Plot"=2, "Plot.Fill/Pt. Color"=u32 6618880, "Plot.Point Style"=11) -> ()  [unwired: 2 in, 2 out]
            n208 = local read "Num Pts Log"() -> (w503:dbl)
            n209 = local read "Sat-Log Slider"() -> (w491:dbl)
            n210 = Unbundle(w506) -> ("[0]"=w505:cluster{dbl[], dbl[]})  [unwired: 8 out]
            n211 = Absolute Value(x=w493) -> (abs(x)=w492:dbl)
            n212 = Unbundle(w505) -> (w494:dbl[], w504:dbl[])
            n213 = Add(x=w491, y=w492) -> (x+y=w488:dbl)
            n214 = Array Subset(array=w494, index=w488, length=w503) -> (w501:dbl[])
            n215 = Array Subset(array=w504, index=w488, length=w503) -> (w502:dbl[])
            n216 = local write "Vg Array-Log-Used"(w501) -> ()
            n217 = local write "IndexLog-Sat"(w488) -> ()
            n218 = Bundle(w501, w502) -> (w487:cluster{dbl[], dbl[]})  [unwired: 1 in]
            n219 = call "STS-Used.vi"("Id Used"=w502, "Vg-Used"=w501) -> ("STS"=w498:dbl)  [unwired: 9 in]
            n220 = local write "Sat Id-Log-Used"(w502) -> ()
            n221 = local read "Re-Calculated Values Cluster"() -> (w500:T9)
            n222 = Bundle By Name(cluster=w500, "STS"=w498) -> (w499:T9)
            n223 = local write "Re-Calculated Values Cluster"(w499) -> ()
            n224 = Build Array (concatenate)(w496, w497, w487) -> (w495:cluster{dbl[], dbl[]}[])
            n225 = local write "Sat-Log"(w495) -> ()
          }
          event "Lin-Log Slider": Value Change {
            n226 = event-data() -> ()  [unwired: 1 in, 5 out]
            n227 = local read "Lin-Log"() -> (w514:cluster{dbl[], dbl[]}[])
            n228 = Decimate 1D Array(w514) -> (w520:cluster{dbl[], dbl[]}[], w521:cluster{dbl[], dbl[]}[])
            n229 = local read "Slider Min"() -> (w517:dbl)
            n230 = Array To Cluster(array=w520) -> (cluster=w527:T19)
            n231 = local read "Num Pts Log"() -> (w524:dbl)
            n232 = property on="Lin-Log" class="XYGraph (strict)"("Active Plot"=2, "Plot.Fill/Pt. Color"=u32 6618880, "Plot.Point Style"=11) -> ()  [unwired: 2 in, 2 out]
            n233 = local read "Lin-Log Slider"() -> (w515:dbl)
            n234 = Unbundle(w527) -> ("[0]"=w526:cluster{dbl[], dbl[]})  [unwired: 8 out]
            n235 = Absolute Value(x=w517) -> (abs(x)=w516:dbl)
            n236 = Unbundle(w526) -> (w518:dbl[], w525:dbl[])
            n237 = Add(x=w515, y=w516) -> (x+y=w513:dbl)
            n238 = Array Subset(array=w518, index=w513, length=w524) -> (w522:dbl[])
            n239 = local write "Lin-Vg Array-Log Used"(w522) -> ()
            n240 = Array Subset(array=w525, index=w513, length=w524) -> (w523:dbl[])
            n241 = local write "IndexLog-Sat"(w513) -> ()
            n242 = Bundle(w522, w523) -> (w512:cluster{dbl[], dbl[]})  [unwired: 1 in]
            n243 = local write "Lin Id-Log Used"(w523) -> ()
            n244 = Build Array (concatenate)(w520, w521, w512) -> (w519:cluster{dbl[], dbl[]}[])
            n245 = local write "Lin-Log"(w519) -> ()
          }
          event "Index Array": Value Change {
            n246 = event-data() -> ()  [unwired: 1 in, 5 out]
            n247 = Strip Path(path=w528) -> (stripped path=w534:path)  [unwired: 1 out]
            n248 = local write "Transfer Folder"(w534) -> ()
            n249 = List Folder(path=w534) -> (filenames=w530:string[])  [unwired: 3 in, 3 out]
            n250 = local read "Index Array"() -> (w529:i32)
            n251 = Path To String(path=w534) -> (string=w535:string)
            n252 = Index Array(array=w530, index=w529) -> (element=w536:string)
            n253 = Concatenate Strings(w535, "\\", w536) -> (w532:string)
            n254 = String To Path(string=w532) -> (path=w531:path)
            n255 = local write "Transfer File"(w531) -> ()
          }
          event "Transfer File": Value Change {
            n256 = event-data() -> ()  [unwired: 1 in, 5 out]
          }
          event "Remove Button": Mouse Down {
            w542 = 0
            n257 = event-data() -> ()  [unwired: 1 in, 5 out]
            n258 = property on="Image Out" class="ImageControl"() -> ("ROI"=w552:T17)  [unwired: 2 in, 2 out]
            n259 = Unbundle(w552) -> ("Global Rectangle"=w543:i32[], "Contours"=w545:T18)
            n260 = Reverse 1D Array(array=w543) -> (reversed array=w544:i32[])
            n261 = Reverse 1D Array(array=w545) -> (reversed array=w546:T18)
            n262 = Delete From Array(array=w544, index=w542) -> (array with subset deleted=w547:i32[])  [unwired: 1 in, 1 out]
            n263 = Delete From Array(array=w546, index=w542) -> (array with subset deleted=w548:T18)  [unwired: 1 in, 1 out]
            n264 = Reverse 1D Array(array=w547) -> (reversed array=w549:i32[])
            n265 = Reverse 1D Array(array=w548) -> (reversed array=w550:T18)
            n266 = Bundle(w549, w550) -> (w551:T20)  [unwired: 1 in]
            n267 = property on="Image Out" class="ImageControl"("ROI"=w551) -> ()  [unwired: 2 in, 2 out]
          }
          event "Undo Button": Mouse Down {
            n268 = event-data() -> ()  [unwired: 1 in, 5 out]
            n269 = invoke on="Image Out" class="ImageControl" method="Clear ROI"() -> ()  [unwired: 3 in, 3 out]
          }
          event "Image Folder": Value Change {
            n270 = event-data() -> ()  [unwired: 1 in, 5 out]
            n271 = local read "Image File"() -> (w557:path)
            n272 = call "Vision Acquisition"("Image Path"=w557) -> ("Image Out"=w558:T8)  [unwired: 25 in, 1 out]
            n273 = local write "Image Preview"(w558) -> ()
            n274 = local write "Image Out"(w558) -> ()
          }
          event "Zoom": Value Change {
            n275 = event-data() -> ()  [unwired: 1 in, 5 out]
            n276 = local read "Zoom"() -> (w562:i32)
            n277 = Bundle("Zoom"=w562, "Zoom"=w562) -> (w561:cluster{"Zoom":i32, "Zoom":i32})  [unwired: 1 in]
            n278 = property on="Image Out" class="ImageControl"("ZoomInteger"=w561) -> ()  [unwired: 2 in, 2 out]
          }
          event "Image Out": Mouse Enter {
            n279 = event-data() -> ()  [unwired: 1 in, 3 out]
            n280 = call "Simulate_Keyboard.vi"("Action"=0, "Virtual Key"=162) -> ()  [unwired: 7 in, 1 out]
          }
          event "Image Out": Mouse Leave {
            n281 = event-data() -> ()  [unwired: 1 in, 3 out]
            n282 = flat-sequence {
              frame #0 {
                n283 = Wait (ms)(milliseconds to wait=10) -> ()  [unwired: 1 out]
              }
              frame #1 {
                n284 = call "Simulate_Keyboard.vi"("Action"=2, "Virtual Key"=162) -> ()  [unwired: 7 in, 1 out]
              }
            }
          }
        }
        n285 = Build Array(0.505025, 0.252522, 0.127742, 0.050345, 0.031129) -> (w113:dbl[])
        n286 = Array Subset(array=w113, index="Magnification", length=1) -> (w115:dbl[])
        n287 = To Double Precision Float(number=w115) -> (double precision float=w116:dbl[])
        n288 = for {
          N: w105 -> [_]
          shift-right: [w199] -> _
          shift-left: w104 -> [w199]
          shift-right: [w175] -> w91
          shift-left: w106 -> [w197]
          tunnel: w116 -> [w196]
          shift-right: [w193] -> _
          shift-left: w117 -> [w195]
          tunnel: w101 -> [w189]
          i -> [w192]
          n289 = Index Array(array=w199, index=w192) -> (element=w208:T21)
          n290 = Unbundle(w208) -> ("Points"=w207:i32[])  [unwired: 2 out]
          n291 = Array To Cluster(array=w207) -> (cluster=w206:T22)
          n292 = Unbundle(w206) -> ("Points[0]"=w188:i32, "Points[1]"=w185:i32, "Points[2]"=w198:i32, "Points[3]"=w204:i32)  [unwired: 5 out]
          n293 = Add(x=w188, y=10) -> (x+y=w186:i32)
          n294 = Subtract(x=w185, y=w204) -> (x-y=w203:i32)
          n295 = Subtract(x=w188, y=w198) -> (x-y=w205:i32)
          n296 = Square(x=w203) -> (x^2=w201:i32)
          n297 = Square(x=w205) -> (x^2=w202:i32)
          n298 = Add(x=w202, y=w201) -> (x+y=w200:i32)
          n299 = Square Root(x=w200) -> (sqrt(x)=w179:dbl)
          n300 = Multiply(x=w179, y=0.5) -> (x*y=w182:dbl)
          n301 = Multiply(x=w179, y=w196) -> (x*y=w178:dbl[])
          n302 = Index Array(array=w178) -> (element=w191:dbl)  [unwired: 1 in]
          n303 = Number To Fractional String(number=w191, precision (6)=0) -> (F-format string=w190:string)  [unwired: 2 in]
          n304 = Build Array (concatenate)(w197, w178) -> (w176:dbl[])
          n305 = Add(x=w182, y=w185) -> (x+y=w184:dbl)
          n306 = Bundle(w186, w184) -> (w194:cluster{i32, dbl})  [unwired: 1 in]
          n307 = call "IMAQ Overlay Text"("BG Color (Transparent)"=u32 0, "Text Color (black)"=u32 16448250, "Font, Size & Style"=w189, "String"=w190, "Origin"=w194, "Image"=w195) -> ("Image Out"=w193:T8)  [unwired: 4 in, 1 out]
          n308 = To Long Integer(number=w176) -> (32bit integer=w175:i32[])
        }
        "Distances" <- w91
        n309 = Add Array Elements(numeric array=w91) -> (sum=w102:i32)
        n310 = local write "Total Width"(w102) -> ()
      }
      frame "Read Data" {
        n311 = call "IMAQ Dispose"("All Images? (No)"=TRUE) -> ()  [unwired: 5 in, 1 out]
        n312 = case shown="True" "Disable Flag" {
          tunnel: w618 -> [_ w643]
          tunnel: [w639 w640] -> w617
          tunnel: w615 -> [w639 _]
          frame False {
          }
          frame True {
            n313 = local read "Transfer Folder"() -> (w642:path)
            n314 = List Folder(path=w642) -> (filenames=w644:string[])  [unwired: 3 in, 3 out]
            n315 = Index Array(array=w644, index=w643) -> (element=w641:string)
            n316 = Build Path(base path=w642, name or relative path=w641) -> (appended path=w640:path)
            n317 = local write "Transfer File"(w640) -> ()
          }
        }
        n318 = call "Recorded Values.vi"("Path"=w617) -> ("Recorded Char"=→"Recorded Values Cluster":T9, "Recorded Prop"=w630:T1, "Fabrication Prop"=w628:T4)  [unwired: 8 in]
        n319 = Strip Path(path=w617) -> (stripped path=w627:path, name=w626:string)
        n320 = local write "Fabrication Prop"(w628) -> ()
        n321 = local write "Recorded Prop"(w630) -> ()
        n322 = Unbundle By Name(w630) -> ("Date Recorded"=→"Date Recorded":string, "Index"=w629:string, "Length"=w623:dbl, "Width"=w622:dbl)  [unwired: 1 out]
        n323 = Unbundle By Name(w630) -> ("Sample Temp"=w632:dbl)
        n324 = Unbundle By Name(w628) -> ("Dielectric (nm)"=w624:dbl, "Comments"=w625:string, "Date Created"=→"Date Created":string)
        n325 = List Folder(path=w627) -> (filenames=w621:string[])  [unwired: 3 in, 3 out]
        n326 = local write "Rec: Dielectric (d)"(w624) -> ()
        n327 = local write "Index"(w629) -> ()
        n328 = local write "Rec: Length"(w623) -> ()
        n329 = local write "Rec: Width"(w622) -> ()
        n330 = Equal To 0?(x=w632) -> (x = 0?=w635:bool)
        n331 = Number To Decimal String(number=w632) -> (decimal integer string=w636:string)  [unwired: 1 in]
        n332 = local write "Comments:"(w625) -> ()
        n333 = Search 1D Array(1D array=w621, element=w626) -> (index of element=w620:i32)  [unwired: 1 in]
        n334 = Equal?(x="", y=w636) -> (x = y?=w634:bool)
        n335 = Index Array(array=w621, index=w620) -> (element=→"Data Name:":string)
        n336 = local write "New: Width"(w622) -> ()
        n337 = local write "New: Length"(w623) -> ()
        n338 = local write "Index Array"(w620) -> ()
        n339 = Or(x=w635, y=w634) -> (x .or. y?=w633:bool)
        n340 = local write "New: Dielectric"(w624) -> ()
        n341 = case shown="True" w633 {
          tunnel: [w645 w646] -> w614
          tunnel: w632 -> [w645 _]
          frame False {
          }
          frame True {
            n342 = local read "Room Temp"() -> (w646:dbl)
          }
        }
        n343 = local write "New: Temp"(w614) -> ()
        n344 = Bundle By Name(cluster=w630, "Sample Temp"=w614) -> (w631:T1)
        n345 = local write "Rec: Temp"(w614) -> ()
        n346 = local write "Recorded Prop"(w631) -> ()
      }
      frame "Calculated Values" {
        n347 = local read "Image Center X"() -> (w648:i32)
        n348 = call "Image from TRF Display.vi"("Image Center X"=w648, "No Image File"=w693, "Image Folder"=w694, "Transfer File"=w663) -> ("Image Preview"=w655:T8, "Image Out"=w656:T8, "Image File"=w657:path, "Image Name"=→"Image Name":string, "ROI File"=w652:path)  [unwired: 3 in]
        n349 = invoke on="Image Out" class="ImageControl" method="Clear ROI"() -> ()  [unwired: 3 in, 3 out]
        n350 = local write "Image File"(w657) -> ()
        n351 = local write "Image Out"(w656) -> ()
        n352 = local write "Image Preview"(w655) -> ()
        n353 = call <vilib>:"Check if File or Folder Exists.vi"("path"=w652) -> ("file or folder exists?"=w653:bool, "dup path"=w654:path)  [unwired: 8 in, 1 out]
        n354 = case shown="True" w653 {
          tunnel: w654 -> [_ w714]
          frame False {
          }
          frame True {
            n355 = Read from Text File(file (use dialog)=w714) -> (text=w718:string)  [unwired: 3 in, 3 out]
            n356 = property on="Image Out" class="ImageControl"() -> ("ROI"=w715:T17)  [unwired: 2 in, 2 out]
            n357 = Unflatten From String(type=w715, binary string=w718) -> (value=w716:T17, error out=w717:errorcluster)  [unwired: 3 in, 1 out]
            n358 = property on="Image Out" class="ImageControl"(error in=w717, "ROI"=w716) -> ()  [unwired: 1 in, 2 out]
          }
        }
        n359 = call "TRF to TSP Plot_09_21_12a_JW.vi"("Transport Graph Properties"="Transport Style Controls", "No Transport File"=w658, "Transport Folder"=w659, "Transfer File"=w663) -> ("Transport"=w664:cluster{ext[], ext[]}[], "Transport File"=→"Transport\nFile":path, "Transport Name"=→"Transport Name:":string)  [unwired: 5 in]
        "Transport" <- w664
        n360 = Array Size(array=w664) -> (size(s)=w662:i32)
        n361 = local read "Image Center X"() -> (w649:i32)
        n362 = for {
          N: w662 -> [_]
          tunnel: "Transport Style Controls" -> [w722]
          i -> [w721]
          n363 = Unbundle By Name(w722) -> ("Transport Line Size"=w719:u16, "Transport Line Color"=w720:u32)
          n364 = property on="Transport" class="XYGraph (strict)"("Active Plot"=w721, "Plot.Plot Color"=w720, "Plot.Line Width"=w719) -> ()  [unwired: 2 in, 2 out]
        }
        n365 = local read "Recorded Prop"() -> (w696:T1)
        n366 = local read "Fabrication Prop"() -> (w703:T4)
        n367 = Bundle("Image Center X"=w649, 0) -> (w651:cluster{"Image Center X":i32, i32})  [unwired: 1 in]
        n368 = property on="Image Out" class="ImageControl"("Image Center Position"=w651) -> ()  [unwired: 2 in, 2 out]
        n369 = local read "Calculated Values Cluster"() -> (w713:T9)
        n370 = call "Mobility-Vt Calculator-File.vi"("NumPts"=w698, "Path"=w663) -> ("Used Points"=w691:T23, "Graph Cluster"=w681:T24, "Lin Vd"=w666:dbl, "Output"=w711:T25)  [unwired: 6 in]
        n371 = call "STS Calculator-File.vi"("NumPts"=w697, "Path"=w663) -> ("Used Points"=w686:T26, "XY Graph-Sat"=w670:cluster{dbl[], dbl[]}[], "XY Graph-Lin"=w667:cluster{dbl[], dbl[]}[], "Ouput"=w706:cluster{"STS-Sat":dbl, "STS-Lin":dbl})  [unwired: 6 in]
        n372 = Unbundle By Name(w703) -> ("Dielectric (nm)"=w701:dbl)
        n373 = Unbundle By Name(w696) -> ("Sample Temp"=w695:dbl)
        n374 = Unbundle By Name(w711) -> ("Mobility-Sat"=w710:dbl, "Vt-Sat"=w702:dbl, "Mobility-Lin"=w709:dbl, "Off I-Sat"=w708:dbl, "On/Off I-Sat"=w707:dbl)  [unwired: 1 out]
        n375 = local write "Lin Vd"(w666) -> ()
        n376 = Unbundle By Name(w706) -> ("STS-Sat"=w700:dbl)  [unwired: 1 out]
        n377 = local write "Sat-Log"(w670) -> ()
        n378 = local write "Lin-Log"(w667) -> ()
        n379 = call "Trap Density_VT.vi"("VT"=w702, "Dielectric"=w701) -> ("Trap Density-VT"=w705:dbl)
        n380 = call "Trap Density_STS.vi"("Temp (T) [K]"=w695, "S.T.S. (S)"=w700, "Dielectric"=w701) -> ("Trap Density (N)"=w704:dbl)  [unwired: 8 in]
        n381 = Bundle By Name(cluster=w713, "Mobility-Sat"=w710, "Moblitity-Lin"=w709, "On/Off"=w707, "Off Current"=w708, "Vt-Sat"=w702, "STS"=w700, "Trap Density-VT"=w705, "Trap Density-STS"=w704) -> (w712:T9)
        n382 = Unbundle By Name(w686) -> ("Sat Vg Used"=w685:dbl[], "Sat Log(Id) Used"=w684:dbl[], "Lin Vg Used"=w683:dbl[], "Lin Log(Id) Used"=w682:dbl[], "STS Index-Sat"=w668:dbl, "STS Index-Lin"=w669:dbl)
        n383 = Unbundle By Name(w691) -> ("Sat Vg Used"=w690:dbl[], "Sat Sqrt(Id) Used"=w689:dbl[], "Lin Vg Used"=w688:dbl[], "Lin Sqrt(Id) Used"=w687:dbl[], "Index-Lin"=w677:dbl, "Index-Sat"=w676:dbl)
        n384 = local write "Vg Array-Log-Used"(w685) -> ()
        n385 = local write "Sat Id-Log-Used"(w684) -> ()
        n386 = local write "Lin-Vg Array-Log Used"(w683) -> ()
        n387 = local write "Lin Id-Log Used"(w682) -> ()
        n388 = local write "IndexLog-Sat"(w668) -> ()
        n389 = local write "Index-Lin"(w669) -> ()
        n390 = local write "Calculated Values Cluster"(w712) -> ()
        n391 = local write "Sat Vg Array-Used"(w690) -> ()
        n392 = local write "Sat Id-Used"(w689) -> ()
        n393 = local write "Lin-Vg Array-Used"(w688) -> ()
        n394 = local write "Lin Id-Used"(w687) -> ()
        n395 = local write "Index-Sat"(w676) -> ()
        n396 = local write "Index-Lin"(w677) -> ()
        n397 = local write "Lin-Log Slider"(w669) -> ()
        n398 = local write "Sat-Log Slider"(w668) -> ()
        n399 = local write "Sat-Trans Slider"(w676) -> ()
        n400 = local write "Lin-Trans Slider"(w677) -> ()
        n401 = Unbundle By Name(w681) -> ("Raw Sat"=w675:cluster{dbl[], dbl[]}[], "Sqrt Sat"=w678:cluster{dbl[], dbl[]}[], "Raw Lin"=w680:cluster{dbl[], dbl[]}[], "Sqrt Lin"=w679:cluster{dbl[], dbl[]}[])
        n402 = Index Array(array=w675) -> (element=w674:cluster{dbl[], dbl[]})  [unwired: 1 in]
        n403 = Unbundle(w674) -> (w673:dbl[])  [unwired: 1 out]
        n404 = Array Max & Min(array=w673) -> (max value=w672:dbl, min value=w671:dbl)  [unwired: 2 out]
        n405 = property on="Sat-Trans Slider" class="Slide (strict)"("Scale.Maximum"=w672, "Scale.Minimum"=w671) -> ()  [unwired: 2 in, 2 out]
        n406 = property on="Lin-Trans Slider" class="Slide (strict)"("Scale.Maximum"=w672, "Scale.Minimum"=w671) -> ()  [unwired: 2 in, 2 out]
        n407 = property on="Sat-Log Slider" class="Slide (strict)"("Scale.Maximum"=w672, "Scale.Minimum"=w671) -> ()  [unwired: 2 in, 2 out]
        n408 = property on="Lin-Log Slider" class="Slide (strict)"("Scale.Maximum"=w672, "Scale.Minimum"=w671) -> ()  [unwired: 2 in, 2 out]
        n409 = local write "Slider Max"(w672) -> ()
        n410 = local write "Slider Min"(w671) -> ()
        n411 = local write "Raw- Sat"(w675) -> ()
        n412 = local write "Raw- Lin"(w680) -> ()
        n413 = local write "Sqrt-Sat"(w678) -> ()
        n414 = local write "Sqrt-Lin"(w679) -> ()
      }
      frame "Re-Calculated Values" {
        n415 = local read "Vg Array-Log-Used"() -> (w731:dbl[])
        n416 = local read "Sat Vg Array-Used"() -> (w739:dbl[])
        n417 = local read "Lin-Vg Array-Used"() -> (w745:dbl[])
        n418 = local read "Sat Id-Log-Used"() -> (w730:dbl[])
        n419 = local read "New: Dielectric"() -> (w743:dbl)
        n420 = local read "New: Dielectric"() -> (w728:dbl)
        n421 = local read "New: Length"() -> (w742:dbl)
        n422 = local read "New: Length"() -> (w738:dbl)
        n423 = local read "New: Width"() -> (w741:dbl)
        n424 = local read "New: Width"() -> (w737:dbl)
        n425 = local read "Lin Id-Used"() -> (w744:dbl[])
        n426 = local read "Sat Id-Used"() -> (w736:dbl[])
        n427 = local read "Re-Calculated Values Cluster"() -> (w747:T9)
        n428 = local read "New: Dielectric"() -> (w727:dbl)
        n429 = local read "New: Temp"() -> (w726:dbl)
        n430 = local read "Lin Vd"() -> (w723:dbl)
        n431 = call "Mobility-Vt-Used Pts_Saturation.vi"("Width"=w737, "Length"=w738, "Dielectric (d)"=w728, "Sat Id Used"=w736, "Vg Used"=w739) -> ("Vt"=w734:dbl, "Mobility"=w735:dbl)  [unwired: 4 in, 1 out]
        n432 = call "STS-Used.vi"("Id Used"=w730, "Vg-Used"=w731) -> ("STS"=w729:dbl)  [unwired: 9 in]
        n433 = call "Mobility-Vt-Used Pts_Linear.vi"("Width"=w741, "Length"=w742, "Vd"=w723, "Dielectric (d)"=w743, "Id Used"=w744, "Vg Used"=w745) -> ("Mobility"=w740:dbl)  [unwired: 3 in, 2 out]
        n434 = call "Trap Density_VT.vi"("VT"=w734, "Dielectric"=w728) -> ("Trap Density-VT"=w733:dbl)
        n435 = call "Trap Density_STS.vi"("Temp (T) [K]"=w726, "S.T.S. (S)"=w729, "Dielectric"=w727) -> ("Trap Density (N)"=w725:dbl)  [unwired: 8 in]
        n436 = Bundle By Name(cluster=w747, "Mobility-Sat"=w735, "Moblitity-Lin"=w740, "Vt-Sat"=w734, "STS"=w729, "Trap Density-VT"=w733, "Trap Density-STS"=w725) -> (w746:T9)
        n437 = local write "Re-Calculated Values Cluster"(w746) -> ()
      }
      frame "Next File" {
        n438 = call "IMAQ Dispose"("All Images? (No)"=TRUE) -> ()  [unwired: 5 in, 1 out]
        n439 = Strip Path(path=w764) -> (stripped path=w755:path, name=w762:string)
        n440 = local write "Transfer Folder"(w755) -> ()
        n441 = List Folder(path=w755) -> (filenames=w749:string[])  [unwired: 3 in, 3 out]
        n442 = Array Size(array=w749) -> (size(s)=w761:i32)
        n443 = Search 1D Array(1D array=w749, element=w762) -> (index of element=w759:i32)  [unwired: 1 in]
        n444 = Decrement(x=w761) -> (x-1=w760:i32)
        n445 = Equal?(x=w760, y=w759) -> (x = y?=w758:bool)
        n446 = case shown="True" w758 {
          tunnel: w751 -> [w766 _]
          tunnel: [w765 0] -> w750
          frame False {
            n447 = Increment(x=w766) -> (x+1=w765:i32)
          }
          frame True {
          }
        }
        n448 = Path To String(path=w755) -> (string=w756:string)
        n449 = Index Array(array=w749, index=w750) -> (element=w757:string)
        n450 = Concatenate Strings(w756, "\\", w757) -> (w753:string)
        n451 = String To Path(string=w753) -> (path=w752:path)
        n452 = local write "Transfer File"(w752) -> ()
      }
      frame "Previous File" {
        n453 = call "IMAQ Dispose"("All Images? (No)"=TRUE) -> ()  [unwired: 5 in, 1 out]
        n454 = Strip Path(path=w775) -> (stripped path=w772:path, name=w783:string)
        n455 = local write "Transfer Folder"(w772) -> ()
        n456 = List Folder(path=w772) -> (filenames=w776:string[])  [unwired: 3 in, 3 out]
        n457 = Array Size(array=w776) -> (size(s)=w770:i32)
        n458 = Search 1D Array(1D array=w776, element=w783) -> (index of element=w782:i32)  [unwired: 1 in]
        n459 = Decrement(x=w770) -> (x-1=w769:i32)
        n460 = Equal To 0?(x=w782) -> (x = 0?=w781:bool)
        n461 = case shown="True" w781 {
          tunnel: w774 -> [w786 _]
          tunnel: [w785 w787] -> w773
          tunnel: w769 -> [_ w787]
          frame False {
            n462 = Decrement(x=w786) -> (x-1=w785:i32)
          }
          frame True {
          }
        }
        n463 = Path To String(path=w772) -> (string=w771:string)
        n464 = Index Array(array=w776, index=w773) -> (element=w780:string)
        n465 = Concatenate Strings(w771, "\\", w780) -> (w778:string)
        n466 = String To Path(string=w778) -> (path=w777:path)
        n467 = local write "Transfer File"(w777) -> ()
      }
      frame "Discard File" {
        n468 = Strip Path(path=w802) -> (stripped path=w797:path, name=w796:string)
        n469 = property on="Disable Flag" class="Bool (strict)"("Value"=TRUE) -> ()  [unwired: 2 in, 2 out]
        n470 = List Folder(path=w797) -> (filenames=w795:string[])  [unwired: 3 in, 3 out]
        n471 = Search 1D Array(1D array=w795, element=w796) -> (index of element=w799:i32)  [unwired: 1 in]
        n472 = call "IMAQ Dispose"("All Images? (No)"=TRUE) -> ()  [unwired: 5 in, 1 out]
        n473 = Strip Path(path=w802) -> (stripped path=w794:path, name=w793:string)
        n474 = String Subset(string=w793, offset (0)=0, length (rest)=1) -> (substring=w790:string)
        n475 = Equal?(x=w790, y="X") -> (x = y?=w788:bool)
        n476 = case shown="False" w788 {
          tunnel: w794 -> [w810 _]
          tunnel: w802 -> [w806 _]
          tunnel: w793 -> [w805 _]
          tunnel: w799 -> [w804 w814]
          tunnel: [w804 w813] -> w798
          frame False {
            n477 = Path To String(path=w810) -> (string=w809:string)
            n478 = Concatenate Strings(w809, "\\", "X_", w805) -> (w808:string)
            n479 = String To Path(string=w808) -> (path=w807:path)
            n480 = Move(source path=w806, 10:w807) -> ()  [unwired: 3 in, 3 out]
          }
          frame True {
            n481 = Increment(x=w814) -> (x+1=w813:i32)
          }
        }
      }
      frame "Save" {
        n482 = stacked-sequence {
          seq-local: [w829 _] -> [_ w1326]
          seq-local: [w828 _] -> [_ w1324]
          tunnel: w821 -> [w830 w1327]
          frame #0 {
            # "Saves each Re-calculated parameter in sequence"
            n483 = stacked-sequence {
              tunnel: [_ _ _ _ _ _ _ _ _ _ _ _ _ w1294] -> w828
              tunnel: w830 -> [w850 _ _ _ _ _ _ _ _ _ _ _ _ _]
              frame #0 {
                n484 = call-poly <vilib>:"Read From Spreadsheet File.vi"("file path (dialog if empty)"=w850) -> ("all rows"=w849:string[][])  [unwired: 6 in, 4 out]
                n485 = Array Size(array=w849) -> (size(s)=w854:i32[])
                n486 = Array Subset(array=w849, index (row)=0, index (col)=0, length (col)=3) -> (w858:string[][])  [unwired: 1 in]
                n487 = Index Array(array=w854, index=0) -> (element=w852:i32)
                n488 = Reshape Array(w858, w852) -> (w851:string[])
                n489 = Search 1D Array(1D array=w851, element="Dielectric (nm):") -> (index of element=w861:i32)  [unwired: 1 in]
                n490 = Equal?(x=w861, y=-1) -> (x = y?=w860:bool)
                n491 = case shown="False" w860 {
                  tunnel: w849 -> [w869 w873]
                  tunnel: w861 -> [w865 _]
                  tunnel: [w864 w873] -> w859
                  frame False {
                    n492 = local read "Rec: Dielectric (d)"() -> (w871:dbl)
                    n493 = Number To Fractional String(number=w871) -> (F-format string=w866:string)  [unwired: 3 in]
                    n494 = Divide(x=w865, y=3) -> (x/y=w868:dbl)
                    n495 = To Word Integer(number=w868) -> (16bit integer=w867:i16)
                    n496 = Replace Array Subset(array=w869, new element=w866, index (row)=w867, index (col)=1) -> (w864:string[][])
                  }
                  frame True {
                  }
                }
                n497 = local write "Save Array"(w859) -> ()
              }
              frame #1 {
                n498 = local read "Save Array"() -> (w875:string[][])
                n499 = Array Size(array=w875) -> (size(s)=w878:i32[])
                n500 = Array Subset(array=w875, index (row)=0, index (col)=0, length (col)=3) -> (w882:string[][])  [unwired: 1 in]
                n501 = Index Array(array=w878, index=0) -> (element=w876:i32)
                n502 = Reshape Array(w882, w876) -> (w874:string[])
                n503 = Search 1D Array(1D array=w874, element="Comments:") -> (index of element=w885:i32)  [unwired: 1 in]
                n504 = Equal?(x=w885, y=-1) -> (x = y?=w884:bool)
                n505 = case shown="False" w884 {
                  tunnel: w875 -> [w893 w896]
                  tunnel: w885 -> [w890 _]
                  tunnel: [w889 w896] -> w883
                  frame False {
                    n506 = local read "Comments:"() -> (w888:string)
                    n507 = Divide(x=w890, y=3) -> (x/y=w892:dbl)
                    n508 = To Word Integer(number=w892) -> (16bit integer=w891:i16)
                    n509 = Replace Array Subset(array=w893, new element=w888, index (row)=w891, index (col)=1) -> (w889:string[][])
                  }
                  frame True {
                  }
                }
                n510 = local write "Save Array"(w883) -> ()
              }
              frame #2 {
                n511 = local read "Save Array"() -> (w898:string[][])
                n512 = Array Size(array=w898) -> (size(s)=w901:i32[])
                n513 = Array Subset(array=w898, index (row)=0, index (col)=0, length (col)=3) -> (w905:string[][])  [unwired: 1 in]
                n514 = Index Array(array=w901, index=0) -> (element=w899:i32)
                n515 = Reshape Array(w905, w899) -> (w897:string[])
                n516 = Search 1D Array(1D array=w897, element="Length (um):") -> (index of element=w908:i32)  [unwired: 1 in]
                n517 = Equal?(x=w908, y=-1) -> (x = y?=w907:bool)
                n518 = case shown="False" w907 {
                  tunnel: w898 -> [w918 w921]
                  tunnel: w908 -> [w915 _]
                  tunnel: [w914 w921] -> w906
                  frame False {
                    n519 = local read "New: Length"() -> (w911:dbl)
                    n520 = Divide(x=w915, y=3) -> (x/y=w917:dbl)
                    n521 = Format Value(format string="%#g", value (0)=w911) -> (output string=w912:string)  [unwired: 1 in]
                    n522 = To Word Integer(number=w917) -> (16bit integer=w916:i16)
                    n523 = Replace Array Subset(array=w918, new element=w912, index (row)=w916, index (col)=1) -> (w914:string[][])
                  }
                  frame True {
                  }
                }
                n524 = local write "Save Array"(w906) -> ()
              }
              frame #3 {
                n525 = local read "Save Array"() -> (w923:string[][])
                n526 = Array Size(array=w923) -> (size(s)=w928:i32[])
                n527 = Array Subset(array=w923, index (row)=0, index (col)=0, length (col)=3) -> (w924:string[][])  [unwired: 1 in]
                n528 = Index Array(array=w928, index=0) -> (element=w930:i32)
                n529 = Reshape Array(w924, w930) -> (w922:string[])
                n530 = Search 1D Array(1D array=w922, element="Width (um):") -> (index of element=w933:i32)  [unwired: 1 in]
                n531 = Equal?(x=w933, y=-1) -> (x = y?=w932:bool)
                n532 = case shown="False" w932 {
                  tunnel: w933 -> [w941 _]
                  tunnel: w923 -> [w940 w946]
                  tunnel: [w939 w946] -> w931
                  frame False {
                    n533 = local read "New: Width"() -> (w936:dbl)
                    n534 = Divide(x=w941, y=3) -> (x/y=w943:dbl)
                    n535 = To Word Integer(number=w943) -> (16bit integer=w942:i16)
                    n536 = Format Value(format string="%#g", value (0)=w936) -> (output string=w937:string)  [unwired: 1 in]
                    n537 = Replace Array Subset(array=w940, new element=w937, index (row)=w942, index (col)=1) -> (w939:string[][])
                  }
                  frame True {
                  }
                }
                n538 = local write "Save Array"(w931) -> ()
              }
              frame #4 {
                w956 = "Sample Temp (K):"
                n539 = local read "Save Array"() -> (w948:string[][])
                n540 = Array Size(array=w948) -> (size(s)=w953:i32[])
                n541 = Array Subset(array=w948, index (row)=0, index (col)=0, length (col)=3) -> (w949:string[][])  [unwired: 1 in]
                n542 = Index Array(array=w953, index=0) -> (element=w955:i32)
                n543 = Reshape Array(w949, w955) -> (w947:string[])
                n544 = Search 1D Array(1D array=w947, element=w956) -> (index of element=w959:i32)  [unwired: 1 in]
                n545 = Equal?(x=w959, y=-1) -> (x = y?=w958:bool)
                n546 = case shown="True" w958 {
                  tunnel: w948 -> [w968 w982]
                  tunnel: w959 -> [w965 _]
                  tunnel: [w964 w981] -> w957
                  tunnel: w947 -> [_ w984]
                  tunnel: w956 -> [_ w971]
                  frame False {
                    n547 = local read "New: Temp"() -> (w962:dbl)
                    n548 = Divide(x=w965, y=3) -> (x/y=w967:dbl)
                    n549 = Format Value(format string="%#g", value (0)=w962) -> (output string=w961:string)  [unwired: 1 in]
                    n550 = To Word Integer(number=w967) -> (16bit integer=w966:i16)
                    n551 = Replace Array Subset(array=w968, new element=w961, index (row)=w966, index (col)=1) -> (w964:string[][])
                  }
                  frame True {
                    n552 = local read "New: Temp"() -> (w973:dbl)
                    n553 = Search 1D Array(1D array=w984, element="Width (um):") -> (index of element=w978:i32)  [unwired: 1 in]
                    n554 = Divide(x=w978, y=3) -> (x/y=w979:dbl)
                    n555 = To Word Integer(number=w979) -> (16bit integer=w977:i16)
                    n556 = Format Value(format string="%#g", value (0)=w973) -> (output string=w972:string)  [unwired: 1 in]
                    n557 = Build Array(w971, w972) -> (w975:string[])
                    n558 = Increment(x=w977) -> (x+1=w976:i16)
                    n559 = Insert Into Array(array=w982, index (row)=w976, new element=w975) -> (w981:string[][])  [unwired: 1 in]
                  }
                }
                n560 = local write "Save Array"(w957) -> ()
              }
              frame #5 {
                w994 = "Mobility-Sat (cm^2/Vs):"
                n561 = local read "Save Array"() -> (w986:string[][])
                n562 = Array Size(array=w986) -> (size(s)=w991:i32[])
                n563 = Array Subset(array=w986, index (row)=0, index (col)=0, length (col)=3) -> (w987:string[][])  [unwired: 1 in]
                n564 = Index Array(array=w991, index=0) -> (element=w993:i32)
                n565 = Reshape Array(w987, w993) -> (w985:string[])
                n566 = Search 1D Array(1D array=w985, element=w994) -> (index of element=w997:i32)  [unwired: 1 in]
                n567 = Equal?(x=w997, y=-1) -> (x = y?=w996:bool)
                n568 = case shown="True" w996 {
                  tunnel: w986 -> [w1007 w1017]
                  tunnel: w997 -> [w1004 _]
                  tunnel: [w1003 w1016] -> w995
                  tunnel: w985 -> [_ w1014]
                  tunnel: w994 -> [_ w1012]
                  frame False {
                    n569 = local read "Re-Calculated Values Cluster"() -> (w1000:T9)
                    n570 = Unbundle By Name(w1000) -> ("Mobility-Sat"=w999:dbl)
                    n571 = Divide(x=w1004, y=3) -> (x/y=w1006:dbl)
                    n572 = To Word Integer(number=w1006) -> (16bit integer=w1005:i16)
                    n573 = Format Value(format string="%#g", value (0)=w999) -> (output string=w1001:string)  [unwired: 1 in]
                    n574 = Replace Array Subset(array=w1007, new element=w1001, index (row)=w1005, index (col)=1) -> (w1003:string[][])
                  }
                  frame True {
                    n575 = local read "Re-Calculated Values Cluster"() -> (w1011:T9)
                    n576 = Unbundle By Name(w1011) -> ("Mobility-Sat"=w1010:dbl)
                    n577 = Search 1D Array(1D array=w1014, element="Mobility (cm^2/Vs):") -> (index of element=w1020:i32)  [unwired: 1 in]
                    n578 = Divide(x=w1020, y=3) -> (x/y=w1021:dbl)
                    n579 = To Word Integer(number=w1021) -> (16bit integer=w1013:i16)
                    n580 = Format Value(format string="%#g", value (0)=w1010) -> (output string=w1015:string)  [unwired: 1 in]
                    n581 = Build Array(w1012, w1015) -> (w1019:string[])
                    n582 = Replace Array Subset(array=w1017, new element=w1019, index (row)=w1013) -> (w1016:string[][])  [unwired: 1 in]
                  }
                }
                n583 = local write "Save Array"(w995) -> ()
              }
              frame #6 {
                w1033 = "Mobility-Lin (cm^2/Vs):"
                n584 = local read "Save Array"() -> (w1024:string[][])
                n585 = Array Size(array=w1024) -> (size(s)=w1030:i32[])
                n586 = Array Subset(array=w1024, index (row)=0, index (col)=0, length (col)=3) -> (w1026:string[][])  [unwired: 1 in]
                n587 = Index Array(array=w1030, index=0) -> (element=w1032:i32)
                n588 = Reshape Array(w1026, w1032) -> (w1025:string[])
                n589 = Search 1D Array(1D array=w1025, element=w1033) -> (index of element=w1036:i32)  [unwired: 1 in]
                n590 = Equal?(x=w1036, y=-1) -> (x = y?=w1035:bool)
                n591 = case shown="True" w1035 {
                  tunnel: w1024 -> [w1046 w1054]
                  tunnel: w1036 -> [w1043 _]
                  tunnel: [w1042 w1053] -> w1034
                  tunnel: w1025 -> [_ w1052]
                  tunnel: w1033 -> [_ w1051]
                  frame False {
                    n592 = local read "Re-Calculated Values Cluster"() -> (w1039:T9)
                    n593 = Unbundle By Name(w1039) -> ("Moblitity-Lin"=w1038:dbl)
                    n594 = Divide(x=w1043, y=3) -> (x/y=w1045:dbl)
                    n595 = To Word Integer(number=w1045) -> (16bit integer=w1044:i16)
                    n596 = Format Value(format string="%#g", value (0)=w1038) -> (output string=w1040:string)  [unwired: 1 in]
                    n597 = Replace Array Subset(array=w1046, new element=w1040, index (row)=w1044, index (col)=1) -> (w1042:string[][])
                  }
                  frame True {
                    n598 = local read "Re-Calculated Values Cluster"() -> (w1050:T9)
                    n599 = Unbundle By Name(w1050) -> ("Moblitity-Lin"=w1049:dbl)
                    n600 = Search 1D Array(1D array=w1052, element="Mobility-Sat (cm^2/Vs):") -> (index of element=w1059:i32)  [unwired: 1 in]
                    n601 = Divide(x=w1059, y=3) -> (x/y=w1060:dbl)
                    n602 = To Word Integer(number=w1060) -> (16bit integer=w1058:i16)
                    n603 = Format Value(format string="%#g", value (0)=w1049) -> (output string=w1063:string)  [unwired: 1 in]
                    n604 = Build Array(w1051, w1063) -> (w1056:string[])
                    n605 = Increment(x=w1058) -> (x+1=w1057:i16)
                    n606 = Insert Into Array(array=w1054, index (row)=w1057, new element=w1056) -> (w1053:string[][])  [unwired: 1 in]
                  }
                }
                n607 = local write "Save Array"(w1034) -> ()
              }
              frame #7 {
                w1073 = "On/Off I-Sat:"
                n608 = local read "Save Array"() -> (w1064:string[][])
                n609 = Array Size(array=w1064) -> (size(s)=w1070:i32[])
                n610 = Array Subset(array=w1064, index (row)=0, index (col)=0, length (col)=3) -> (w1066:string[][])  [unwired: 1 in]
                n611 = Index Array(array=w1070, index=0) -> (element=w1072:i32)
                n612 = Reshape Array(w1066, w1072) -> (w1065:string[])
                n613 = Search 1D Array(1D array=w1065, element=w1073) -> (index of element=w1076:i32)  [unwired: 1 in]
                n614 = Equal?(x=w1076, y=-1) -> (x = y?=w1075:bool)
                n615 = case shown="True" w1075 {
                  tunnel: w1064 -> [w1086 w1095]
                  tunnel: w1076 -> [w1083 _]
                  tunnel: [w1082 w1096] -> w1074
                  tunnel: w1065 -> [_ w1093]
                  tunnel: w1073 -> [_ w1091]
                  frame False {
                    n616 = local read "Calculated Values Cluster"() -> (w1079:T9)
                    n617 = Divide(x=w1083, y=3) -> (x/y=w1085:dbl)
                    n618 = Unbundle By Name(w1079) -> ("On/Off"=w1078:dbl)
                    n619 = To Word Integer(number=w1085) -> (16bit integer=w1084:i16)
                    n620 = Format Value(format string="%#g", value (0)=w1078) -> (output string=w1080:string)  [unwired: 1 in]
                    n621 = Replace Array Subset(array=w1086, new element=w1080, index (row)=w1084, index (col)=1) -> (w1082:string[][])
                  }
                  frame True {
                    n622 = local read "Calculated Values Cluster"() -> (w1090:T9)
                    n623 = Unbundle By Name(w1090) -> ("On/Off"=w1089:dbl)
                    n624 = Search 1D Array(1D array=w1093, element="On/Off Current:") -> (index of element=w1099:i32)  [unwired: 1 in]
                    n625 = Divide(x=w1099, y=3) -> (x/y=w1100:dbl)
                    n626 = To Word Integer(number=w1100) -> (16bit integer=w1092:i16)
                    n627 = Format Value(format string="%#g", value (0)=w1089) -> (output string=w1094:string)  [unwired: 1 in]
                    n628 = Build Array(w1091, w1094) -> (w1098:string[])
                    n629 = Replace Array Subset(array=w1095, new element=w1098, index (row)=w1092) -> (w1096:string[][])  [unwired: 1 in]
                  }
                }
                n630 = local write "Save Array"(w1074) -> ()
              }
              frame #8 {
                w1112 = "Off I-Sat (A):"
                n631 = local read "Save Array"() -> (w1103:string[][])
                n632 = Array Size(array=w1103) -> (size(s)=w1109:i32[])
                n633 = Array Subset(array=w1103, index (row)=0, index (col)=0, length (col)=3) -> (w1105:string[][])  [unwired: 1 in]
                n634 = Index Array(array=w1109, index=0) -> (element=w1111:i32)
                n635 = Reshape Array(w1105, w1111) -> (w1104:string[])
                n636 = Search 1D Array(1D array=w1104, element=w1112) -> (index of element=w1115:i32)  [unwired: 1 in]
                n637 = Equal?(x=w1115, y=-1) -> (x = y?=w1114:bool)
                n638 = case shown="True" w1114 {
                  tunnel: w1103 -> [w1125 w1133]
                  tunnel: w1115 -> [w1122 _]
                  tunnel: [w1121 w1132] -> w1113
                  tunnel: w1104 -> [_ w1131]
                  tunnel: w1112 -> [_ w1130]
                  frame False {
                    # "New Data File"
                    n639 = local read "Calculated Values Cluster"() -> (w1118:T9)
                    n640 = Unbundle By Name(w1118) -> ("Off Current"=w1117:dbl)
                    n641 = Divide(x=w1122, y=3) -> (x/y=w1124:dbl)
                    n642 = Format Value(format string="%#g", value (0)=w1117) -> (output string=w1119:string)  [unwired: 1 in]
                    n643 = To Word Integer(number=w1124) -> (16bit integer=w1123:i16)
                    n644 = Replace Array Subset(array=w1125, new element=w1119, index (row)=w1123, index (col)=1) -> (w1121:string[][])
                  }
                  frame True {
                    # "Old Data File"
                    n645 = local read "Calculated Values Cluster"() -> (w1129:T9)
                    n646 = Unbundle By Name(w1129) -> ("Off Current"=w1128:dbl)
                    n647 = Search 1D Array(1D array=w1131, element="On/Off I-Sat:") -> (index of element=w1138:i32)  [unwired: 1 in]
                    n648 = Divide(x=w1138, y=3) -> (x/y=w1139:dbl)
                    n649 = To Word Integer(number=w1139) -> (16bit integer=w1137:i16)
                    n650 = Format Value(format string="%#g", value (0)=w1128) -> (output string=w1142:string)  [unwired: 1 in]
                    n651 = Build Array(w1130, w1142) -> (w1135:string[])
                    n652 = Increment(x=w1137) -> (x+1=w1136:i16)
                    n653 = Insert Into Array(array=w1133, index (row)=w1136, new element=w1135) -> (w1132:string[][])  [unwired: 1 in]
                  }
                }
                n654 = local write "Save Array"(w1113) -> ()
              }
              frame #9 {
                w1144 = "Vt-Sat (V):"
                n655 = local read "Save Array"() -> (w1145:string[][])
                n656 = Array Size(array=w1145) -> (size(s)=w1150:i32[])
                n657 = Array Subset(array=w1145, index (row)=0, index (col)=0, length (col)=3) -> (w1146:string[][])  [unwired: 1 in]
                n658 = Index Array(array=w1150, index=0) -> (element=w1152:i32)
                n659 = Reshape Array(w1146, w1152) -> (w1143:string[])
                n660 = Search 1D Array(1D array=w1143, element=w1144) -> (index of element=w1155:i32)  [unwired: 1 in]
                n661 = Equal?(x=w1155, y=-1) -> (x = y?=w1154:bool)
                n662 = case shown="True" w1154 {
                  tunnel: w1145 -> [w1164 w1174]
                  tunnel: w1155 -> [w1160 _]
                  tunnel: [w1159 w1173] -> w1153
                  tunnel: w1144 -> [_ w1172]
                  tunnel: w1143 -> [_ w1171]
                  frame False {
                    n663 = local read "Re-Calculated Values Cluster"() -> (w1158:T9)
                    n664 = Unbundle By Name(w1158) -> ("Vt-Sat"=w1157:dbl)
                    n665 = Divide(x=w1160, y=3) -> (x/y=w1163:dbl)
                    n666 = To Word Integer(number=w1163) -> (16bit integer=w1162:i16)
                    n667 = Number To Fractional String(number=w1157) -> (F-format string=w1161:string)  [unwired: 3 in]
                    n668 = Replace Array Subset(array=w1164, new element=w1161, index (row)=w1162, index (col)=1) -> (w1159:string[][])
                  }
                  frame True {
                    n669 = local read "Re-Calculated Values Cluster"() -> (w1168:T9)
                    n670 = Unbundle By Name(w1168) -> ("Vt-Sat"=w1167:dbl)
                    n671 = Search 1D Array(1D array=w1171, element="Threshold V (V):") -> (index of element=w1170:i32)  [unwired: 1 in]
                    n672 = Divide(x=w1170, y=3) -> (x/y=w1177:dbl)
                    n673 = To Word Integer(number=w1177) -> (16bit integer=w1169:i16)
                    n674 = Format Value(format string="%#g", value (0)=w1167) -> (output string=w1180:string)  [unwired: 1 in]
                    n675 = Build Array(w1172, w1180) -> (w1176:string[])
                    n676 = Replace Array Subset(array=w1174, new element=w1176, index (row)=w1169) -> (w1173:string[][])  [unwired: 1 in]
                  }
                }
                n677 = local write "Save Array"(w1153) -> ()
              }
              frame #10 {
                n678 = disable-structure shown="Disabled" {
                  frame Disabled {
                    n679 = local read "Save Array"() -> (w1181:string[][])
                    n680 = Array Size(array=w1181) -> (size(s)=w1187:i32[])
                    n681 = Array Subset(array=w1181, index (row)=0, index (col)=0, length (col)=3) -> (w1183:string[][])  [unwired: 1 in]
                    n682 = Index Array(array=w1187, index=0) -> (element=w1189:i32)
                    n683 = Reshape Array(w1183, w1189) -> (w1182:string[])
                    n684 = Search 1D Array(1D array=w1182, element="VT-Lin (V):") -> (index of element=w1192:i32)  [unwired: 1 in]
                    n685 = Equal?(x=w1192, y=-1) -> (x = y?=w1191:bool)
                    n686 = case shown="False" w1191 {
                      tunnel: w1181 -> [w1201 w1204]
                      tunnel: w1192 -> [w1198 _]
                      tunnel: [w1197 w1204] -> w1190
                      frame False {
                        n687 = Divide(x=w1198, y=3) -> (x/y=w1200:dbl)
                        n688 = To Word Integer(number=w1200) -> (16bit integer=w1199:i16)
                        n689 = Format Value(format string="%#g") -> (output string=w1195:string)  [unwired: 2 in]
                        n690 = Replace Array Subset(array=w1201, new element=w1195, index (row)=w1199, index (col)=1) -> (w1197:string[][])
                      }
                      frame True {
                      }
                    }
                    n691 = local write "Save Array"(w1190) -> ()
                  }
                  frame Enabled {
                  }
                }
              }
              frame #11 {
                w1205 = "STS-Sat (V/decade):"
                n692 = local read "Save Array"() -> (w1207:string[][])
                n693 = Array Size(array=w1207) -> (size(s)=w1212:i32[])
                n694 = Array Subset(array=w1207, index (row)=0, index (col)=0, length (col)=3) -> (w1208:string[][])  [unwired: 1 in]
                n695 = Index Array(array=w1212, index=0) -> (element=w1214:i32)
                n696 = Reshape Array(w1208, w1214) -> (w1206:string[])
                n697 = Search 1D Array(1D array=w1206, element=w1205) -> (index of element=w1217:i32)  [unwired: 1 in]
                n698 = Equal?(x=w1217, y=-1) -> (x = y?=w1216:bool)
                n699 = case shown="True" w1216 {
                  tunnel: w1207 -> [w1227 w1235]
                  tunnel: w1217 -> [w1224 _]
                  tunnel: [w1223 w1236] -> w1215
                  tunnel: w1206 -> [_ w1234]
                  tunnel: w1205 -> [_ w1233]
                  frame False {
                    # "Current Data File"
                    n700 = local read "Re-Calculated Values Cluster"() -> (w1219:T9)
                    n701 = Unbundle By Name(w1219) -> ("STS"=w1220:dbl)
                    n702 = Divide(x=w1224, y=3) -> (x/y=w1226:dbl)
                    n703 = To Word Integer(number=w1226) -> (16bit integer=w1225:i16)
                    n704 = Format Value(format string="%#g", value (0)=w1220) -> (output string=w1221:string)  [unwired: 1 in]
                    n705 = Replace Array Subset(array=w1227, new element=w1221, index (row)=w1225, index (col)=1) -> (w1223:string[][])
                  }
                  frame True {
                    # "Old Data File"
                    n706 = local read "Re-Calculated Values Cluster"() -> (w1230:T9)
                    n707 = Unbundle By Name(w1230) -> ("STS"=w1231:dbl)
                    n708 = Search 1D Array(1D array=w1234, element="S.T.S. (V/decade):") -> (index of element=w1239:i32)  [unwired: 1 in]
                    n709 = Divide(x=w1239, y=3) -> (x/y=w1240:dbl)
                    n710 = To Word Integer(number=w1240) -> (16bit integer=w1232:i16)
                    n711 = Format Value(format string="%#g", value (0)=w1231) -> (output string=w1243:string)  [unwired: 1 in]
                    n712 = Build Array(w1233, w1243) -> (w1238:string[])
                    n713 = Replace Array Subset(array=w1235, new element=w1238, index (row)=w1232) -> (w1236:string[][])  [unwired: 1 in]
                  }
                }
                n714 = local write "Save Array"(w1215) -> ()
              }
              frame #12 {
                w1244 = "Trap Density-VT (Traps/Vcm^2):"
                n715 = local read "Save Array"() -> (w1246:string[][])
                n716 = Array Size(array=w1246) -> (size(s)=w1251:i32[])
                n717 = Array Subset(array=w1246, index (row)=0, index (col)=0, length (col)=3) -> (w1247:string[][])  [unwired: 1 in]
                n718 = Index Array(array=w1251, index=0) -> (element=w1253:i32)
                n719 = Reshape Array(w1247, w1253) -> (w1245:string[])
                n720 = Search 1D Array(1D array=w1245, element=w1244) -> (index of element=w1256:i32)  [unwired: 1 in]
                n721 = Equal?(x=w1256, y=-1) -> (x = y?=w1255:bool)
                n722 = case shown="True" w1255 {
                  tunnel: w1246 -> [w1266 w1273]
                  tunnel: w1256 -> [w1262 _]
                  tunnel: [w1261 w1274] -> w1254
                  tunnel: w1245 -> [_ w1272]
                  tunnel: w1244 -> [_ w1271]
                  frame False {
                    n723 = local read "Re-Calculated Values Cluster"() -> (w1259:T9)
                    n724 = Unbundle By Name(w1259) -> ("Trap Density-VT"=w1258:dbl)
                    n725 = Divide(x=w1262, y=3) -> (x/y=w1265:dbl)
                    n726 = To Word Integer(number=w1265) -> (16bit integer=w1264:i16)
                    n727 = Format Value(format string="%#g", value (0)=w1258) -> (output string=w1263:string)  [unwired: 1 in]
                    n728 = Replace Array Subset(array=w1266, new element=w1263, index (row)=w1264, index (col)=1) -> (w1261:string[][])
                  }
                  frame True {
                    n729 = local read "Re-Calculated Values Cluster"() -> (w1270:T9)
                    n730 = Unbundle By Name(w1270) -> ("Trap Density-VT"=w1269:dbl)
                    n731 = Search 1D Array(1D array=w1272, element="STS-Sat (V/decade):") -> (index of element=w1279:i32)  [unwired: 1 in]
                    n732 = Divide(x=w1279, y=3) -> (x/y=w1278:dbl)
                    n733 = To Word Integer(number=w1278) -> (16bit integer=w1280:i16)
                    n734 = Format Value(format string="%#g", value (0)=w1269) -> (output string=w1275:string)  [unwired: 1 in]
                    n735 = Build Array(w1271, w1275) -> (w1282:string[])
                    n736 = Increment(x=w1280) -> (x+1=w1281:i16)
                    n737 = Insert Into Array(array=w1273, index (row)=w1281, new element=w1282) -> (w1274:string[][])  [unwired: 1 in]
                  }
                }
                n738 = local write "Save Array"(w1254) -> ()
              }
              frame #13 {
                w1284 = "Trap Density-STS (Traps/Vcm^2):"
                n739 = local read "Save Array"() -> (w1286:string[][])
                n740 = Array Size(array=w1286) -> (size(s)=w1291:i32[])
                n741 = Array Subset(array=w1286, index (row)=0, index (col)=0, length (col)=3) -> (w1287:string[][])  [unwired: 1 in]
                n742 = Index Array(array=w1291, index=0) -> (element=w1293:i32)
                n743 = Reshape Array(w1287, w1293) -> (w1285:string[])
                n744 = Search 1D Array(1D array=w1285, element=w1284) -> (index of element=w1296:i32)  [unwired: 1 in]
                n745 = Equal?(x=w1296, y=-1) -> (x = y?=w1295:bool)
                n746 = case shown="True" w1295 {
                  tunnel: w1286 -> [w1306 w1313]
                  tunnel: w1296 -> [w1303 _]
                  tunnel: [w1302 w1314] -> w1294
                  tunnel: w1285 -> [_ w1312]
                  tunnel: w1284 -> [_ w1311]
                  frame False {
                    n747 = local read "Re-Calculated Values Cluster"() -> (w1299:T9)
                    n748 = Unbundle By Name(w1299) -> ("Trap Density-STS"=w1298:dbl)
                    n749 = Divide(x=w1303, y=3) -> (x/y=w1305:dbl)
                    n750 = To Word Integer(number=w1305) -> (16bit integer=w1304:i16)
                    n751 = Format Value(format string="%#g", value (0)=w1298) -> (output string=w1300:string)  [unwired: 1 in]
                    n752 = Replace Array Subset(array=w1306, new element=w1300, index (row)=w1304, index (col)=1) -> (w1302:string[][])
                  }
                  frame True {
                    n753 = local read "Re-Calculated Values Cluster"() -> (w1310:T9)
                    n754 = Unbundle By Name(w1310) -> ("Trap Density-STS"=w1309:dbl)
                    n755 = Search 1D Array(1D array=w1312, element="Trap Density-VT (Traps/Vcm^2):") -> (index of element=w1319:i32)  [unwired: 1 in]
                    n756 = Divide(x=w1319, y=3) -> (x/y=w1320:dbl)
                    n757 = To Word Integer(number=w1320) -> (16bit integer=w1318:i16)
                    n758 = Format Value(format string="%#g", value (0)=w1309) -> (output string=w1323:string)  [unwired: 1 in]
                    n759 = Build Array(w1311, w1323) -> (w1316:string[])
                    n760 = Increment(x=w1318) -> (x+1=w1317:i16)
                    n761 = Insert Into Array(array=w1313, index (row)=w1317, new element=w1316) -> (w1314:string[][])  [unwired: 1 in]
                  }
                }
                n762 = local write "Save Array"(w1294) -> ()
              }
            }
            n763 = local read "New: Temp"() -> (w831:dbl)
            n764 = local read "New: Width"() -> (w832:dbl)
            n765 = local read "New: Length"() -> (w834:dbl)
            n766 = local read "Index"() -> (w833:string)
            n767 = To Single Precision Float(number=w831) -> (single precision float=w848:sgl)
            n768 = Number To Decimal String(number=w848) -> (decimal integer string=w843:string)  [unwired: 1 in]
            n769 = To Single Precision Float(number=w832) -> (single precision float=w847:sgl)
            n770 = To Single Precision Float(number=w834) -> (single precision float=w846:sgl)
            n771 = Strip Path(path=w830) -> (stripped path=w835:path)  [unwired: 1 out]
            n772 = Number To Decimal String(number=w846) -> (decimal integer string=w841:string)  [unwired: 1 in]
            n773 = Number To Decimal String(number=w847) -> (decimal integer string=w840:string)  [unwired: 1 in]
            n774 = Concatenate Strings("_", w843, "K") -> (w845:string)
            n775 = call "Build Text"("Temp"=w845, "Index"=w833, "Length"=w841, "Width"=w840) -> ("Result"=w839:string)  [unwired: 10 in, 1 out]
            n776 = Path To String(path=w835) -> (string=w837:string)
            n777 = Concatenate Strings(w837, "\\", w839) -> (w838:string)
            n778 = String To Path(string=w838) -> (path=w829:path)
          }
          frame #1 {
            n779 = flat-sequence {
              tunnel: w1327 -> [w1329]
              tunnel: w1326 -> [w1328]
              tunnel: [w1328] -> w1325
              tunnel: w1325 -> [w1335]
              tunnel: w1324 -> [w1334]
              frame #0 {
                n780 = Equal?(x=w1329, y=w1328) -> (x = y?=w1330:bool)
                n781 = case shown="False" w1330 {
                  tunnel: w1329 -> [w1333 _]
                  tunnel: w1328 -> [w1332 _]
                  frame False {
                    n782 = Move(source path=w1333, 9:TRUE, 10:w1332) -> ()  [unwired: 2 in, 3 out]
                  }
                  frame True {
                  }
                }
              }
              frame #1 {
                n783 = local write "Transfer File"(w1335) -> ()
                n784 = call-poly <vilib>:"Write To Spreadsheet File.vi"("2D data"=w1334, "file path (dialog if empty)"=w1335) -> ()  [unwired: 6 in, 1 out]
              }
            }
          }
        }
        n785 = local read "Save Next?"() -> (w815:bool)
        n786 = Cluster To Array(cluster=w820) -> (array=w819:bool[])
        n787 = Boolean Array To Number(Boolean array=w819) -> (number=w818:u32)
        n788 = Equal To 0?(x=w818) -> (x = 0?=w817:bool)
        n789 = case shown="True" w817 {
          tunnel: [MegaAwesome_States."Read Data" w827] -> w816
          tunnel: w815 -> [_ w824]
          frame False {
          }
          frame True {
            n790 = Select(t=MegaAwesome_States."Next File", s=w824, f=MegaAwesome_States."No Event") -> (s? t:f=w827:T2)
          }
        }
      }
      frame "Exit" {
        n791 = disable-structure shown="Disabled" {
          disable-tunnel: [w1339 _] -> _
          disable-tunnel: [w1338 _] -> _
          frame Disabled {
            n792 = flat-sequence {
              tunnel: [w1348] -> w1339
              tunnel: [w1348] -> w1338
              frame #0 {
                w1347 = FALSE
                n793 = property on="Next File" class="Bool (strict)"("Value"=w1347) -> (error out=w1342:errorcluster)  [unwired: 2 in, 1 out]
                n794 = property on="Previous File" class="Bool (strict)"(error in=w1342, "Value"=w1347) -> (error out=w1343:errorcluster)  [unwired: 1 in, 1 out]
                n795 = Request Deallocation(TRUE) -> ()
                n796 = property on="Save" class="Bool (strict)"(error in=w1343, "Value"=w1347) -> (error out=w1344:errorcluster)  [unwired: 1 in, 1 out]
                n797 = property on="Export" class="Bool (strict)"("Value"=w1347) -> ()  [unwired: 2 in, 2 out]
                n798 = property on="Save Next" class="Bool (strict)"(error in=w1344, "Value"=w1347) -> (error out=w1345:errorcluster)  [unwired: 1 in, 1 out]
                n799 = property on="Discard" class="Bool (strict)"(error in=w1345, "Value"=w1347) -> (error out=w1346:errorcluster)  [unwired: 1 in, 1 out]
                n800 = property on="Save Lines" class="Bool (strict)"(error in=w1346, "Value"=w1347) -> ()  [unwired: 1 in, 2 out]
                n801 = property on="Close" class="Bool (strict)"("Value"=w1347) -> ()  [unwired: 2 in, 2 out]
                n802 = property on="Disable Flag" class="Bool (strict)"("Value"=w1347) -> ()  [unwired: 2 in, 2 out]
                n803 = call "IMAQ Dispose"("All Images? (No)"=TRUE) -> ()  [unwired: 5 in, 1 out]
              }
              frame #1 {
                w1348 = MegaAwesome_States."Exit"
              }
            }
          }
          frame Enabled {
          }
        }
        n804 = event shown="[0] Application Instance Close?" {
          selector: _ -> [_]
          dyn-events: _ -> [_]
          timeout: _ -> [_]
          event Application Instance Close? {
            n805 = event-data() -> ()  [unwired: 1 in, 4 out]
            n806 = event-data("Discard?"=TRUE) -> ()  [unwired: 2 in, 1 out]
          }
        }
      }
      frame "Save Lines" {
        n807 = Build Path(base path=w1351, name or relative path="ROI") -> (appended path=w1354:path)
        n808 = call <vilib>:"Check if File or Folder Exists.vi"("path"=w1354) -> ("file or folder exists?"=w1352:bool, "dup path"=w1355:path)  [unwired: 8 in, 1 out]
        n809 = case shown="False" w1352 {
          tunnel: w1355 -> [w1363 w1364]
          tunnel: [w1362 w1364] -> w1359
          frame False {
            n810 = Create Folder(path (use dialog)=w1363) -> (created path=w1362:path)  [unwired: 2 in, 2 out]
          }
          frame True {
          }
        }
        n811 = local read "Index"() -> (w1350:string)
        n812 = property on="Image Out" class="ImageControl"() -> ("ROI"=w1356:T17)  [unwired: 2 in, 2 out]
        n813 = Build Path(base path=w1359, name or relative path=w1350) -> (appended path=w1358:path)
        n814 = Flatten To String(anything=w1356) -> (data string=w1357:string)  [unwired: 3 in, 2 out]
        n815 = Write to Text File(file (use dialog)=w1358, text=w1357) -> ()  [unwired: 2 in, 3 out]
      }
      frame "Export" {
        n816 = flat-sequence {
          tunnel: ["Independant Variable:"] -> w1365
          tunnel: w1366 -> [w1422]
          tunnel: w1365 -> [w1421]
          frame #0 {
            n817 = stacked-sequence {
              tunnel: "Independant Variable:" -> [w1370 w1375 w1380 w1385 w1390 w1395 w1400 w1405 w1410 w1415]
              frame #0 {
                n818 = Equal?(x=w1370, y="Length (um):") -> (x = y?=w1371:bool)
                n819 = case shown="True" w1371 {
                  frame False {
                  }
                  frame True {
                    n820 = local write "X Axis Display Type"("1") -> ()
                    n821 = local write "Opj X Axis"("2") -> ()
                  }
                }
              }
              frame #1 {
                n822 = Equal?(x=w1375, y="Sample Temp (K):") -> (x = y?=w1376:bool)
                n823 = case shown="True" w1376 {
                  frame False {
                  }
                  frame True {
                    n824 = local write "X Axis Display Type"("1") -> ()
                    n825 = local write "Opj X Axis"("1") -> ()
                  }
                }
              }
              frame #2 {
                n826 = Equal?(x=w1380, y="Mobility-Sat (cm^2/Vs):") -> (x = y?=w1381:bool)
                n827 = case shown="True" w1381 {
                  frame False {
                  }
                  frame True {
                    n828 = local write "X Axis Display Type"("2") -> ()
                    n829 = local write "Opj X Axis"("2") -> ()
                  }
                }
              }
              frame #3 {
                n830 = Equal?(x=w1385, y="Mobility-Lin (cm^2/Vs):") -> (x = y?=w1386:bool)
                n831 = case shown="True" w1386 {
                  frame False {
                  }
                  frame True {
                    n832 = local write "X Axis Display Type"("2") -> ()
                    n833 = local write "Opj X Axis"("2") -> ()
                  }
                }
              }
              frame #4 {
                n834 = Equal?(x=w1390, y="On/Off I-Sat:") -> (x = y?=w1391:bool)
                n835 = case shown="True" w1391 {
                  frame False {
                  }
                  frame True {
                    n836 = local write "X Axis Display Type"("2") -> ()
                    n837 = local write "Opj X Axis"("2") -> ()
                  }
                }
              }
              frame #5 {
                n838 = Equal?(x=w1395, y="Off I-Sat (A):") -> (x = y?=w1396:bool)
                n839 = case shown="True" w1396 {
                  frame False {
                  }
                  frame True {
                    n840 = local write "X Axis Display Type"("2") -> ()
                    n841 = local write "Opj X Axis"("2") -> ()
                  }
                }
              }
              frame #6 {
                n842 = Equal?(x=w1400, y="Vt-Sat (V):") -> (x = y?=w1401:bool)
                n843 = case shown="True" w1401 {
                  frame False {
                  }
                  frame True {
                    n844 = local write "X Axis Display Type"("1") -> ()
                    n845 = local write "Opj X Axis"("1") -> ()
                  }
                }
              }
              frame #7 {
                n846 = Equal?(x=w1405, y="STS-Sat (V/decade):") -> (x = y?=w1406:bool)
                n847 = case shown="True" w1406 {
                  frame False {
                  }
                  frame True {
                    n848 = local write "X Axis Display Type"("1") -> ()
                    n849 = local write "Opj X Axis"("1") -> ()
                  }
                }
              }
              frame #8 {
                n850 = Equal?(x=w1410, y="Trap Density-VT (Traps/Vcm^2):") -> (x = y?=w1411:bool)
                n851 = case shown="True" w1411 {
                  frame False {
                  }
                  frame True {
                    n852 = local write "X Axis Display Type"("2") -> ()
                    n853 = local write "Opj X Axis"("2") -> ()
                  }
                }
              }
              frame #9 {
                n854 = Equal?(x=w1415, y="Trap Density-STS (Traps/Vcm^2):") -> (x = y?=w1416:bool)
                n855 = case shown="True" w1416 {
                  frame False {
                  }
                  frame True {
                    n856 = local write "X Axis Display Type"("2") -> ()
                    n857 = local write "Opj X Axis"("2") -> ()
                  }
                }
              }
            }
          }
          frame #1 {
            n858 = local read "Transfer Folder"() -> (w1426:path)
            n859 = Build Path(base path=w1426, name or relative path="Stats") -> (appended path=w1427:path)
            n860 = call <vilib>:"Check if File or Folder Exists.vi"("path"=w1427) -> ("file or folder exists?"=w1441:bool, "dup path"=w1440:path)  [unwired: 8 in, 1 out]
            n861 = call <userlib>:"OA_ConnectToOrigin.vi"() -> ("error out"=w1438:errorcluster, "Origin.IOApplication"=w1439:refnum<k7>)  [unwired: 8 in]
            n862 = case shown="False" w1441 {
              tunnel: w1440 -> [w1614 w1615]
              tunnel: [w1613 w1615] -> w1425
              frame False {
                n863 = Create Folder(path (use dialog)=w1614) -> (created path=w1613:path)  [unwired: 2 in, 2 out]
              }
              frame True {
              }
            }
            n864 = call "File Dialog"("start path"=w1427) -> ("selected path"=w1429:path)  [unwired: 11 in, 3 out]
            n865 = call <userlib>:"OA_Load.vi"("error in (no error)"=w1438, "Path"=w1422, "Origin.IOApplication"=w1439) -> ("error out"=w1436:errorcluster, "Origin.IOApplication"=w1437:refnum<k7>)  [unwired: 1 out]
            n866 = call "OAExecute.vi"("script"="document -m 3;", "Error IO"=w1436, "Origin.IOApplication"=w1437) -> ("Error IO Out"=w1434:errorcluster, "Origin.IOApplication"=w1435:refnum<k7>)  [unwired: 1 in, 1 out]
            n867 = stacked-sequence {
              tunnel: w1426 -> [w1452 w1482 w1494 w1516 w1536 w1557 w1578 w1601]
              tunnel: w1425 -> [w1453 w1481 w1495 w1515 w1537 w1558 w1579 w1602]
              tunnel: w1435 -> [w1455 w1479 w1497 w1518 w1539 w1560 w1581 w1604]
              tunnel: w1434 -> [w1454 w1480 w1496 w1517 w1538 w1559 w1580 w1603]
              tunnel: [_ _ _ _ _ _ _ w1599] -> w1424
              tunnel: [_ _ _ _ _ _ _ w1600] -> w1423
              tunnel: w1421 -> [w1451 w1472 w1493 w1514 w1535 w1556 w1577 w1598]
              frame #0 {
                n868 = local read "X Axis Display Type"() -> (w1443:string)
                n869 = local read "Opj X Axis"() -> (w1448:string)
                n870 = Concatenate Strings("window -a MOBLGraph;\nlayer.x.type=", w1448, "; layer.x.label.numFormat = ", w1443, "; Y3 = 1; X3 = 1;", "window -a MOBLTable;\nwindow -s TV;") -> (w1446:string)
                n871 = call "Param_Analysis_7_24b_JW.vi"("Independant Variable"=w1451, "error in (no error)"=w1454, "Data Folder"=w1452, "Parameter String"="Mobility-Lin (cm^2/Vs):", "Parameter Name"="Mobility-Lin", "Stats Folder"=w1453) -> ("error out"=w1457:errorcluster, "Output Array"=w1459:string[][], "Variables"=w1450:T27)  [unwired: 2 in, 1 out]
                n872 = call "Origin_Export_7_27a_JW.vi"("Input Conditions"=w1450, "Analysis Array"=w1459, "error in (no error)"=w1457, "Parameter Worksheet Name"="[MOBLTable]Mobilities", "Parameter Folder Script"="pe_cd \"Mobility-Lin\";", "Origin.IOApplication"=w1455) -> ("error out"=w1456:errorcluster, "reference out"=w1458:refnum<k7>)  [unwired: 3 in, 1 out]
                n873 = call "OAExecute.vi"("script"=w1446, "Error IO"=w1456, "Origin.IOApplication"=w1458) -> ()  [unwired: 1 in, 3 out]
              }
              frame #1 {
                n874 = local read "X Axis Display Type"() -> (w1464:string)
                n875 = local read "Opj X Axis"() -> (w1469:string)
                n876 = Concatenate Strings("window -a MOBSGraph;\nlayer.x.type=", w1469, "; layer.x.label.numFormat = ", w1464, "; Y3 = 1; X3 = 1;", "window -a MOBSTable;\nwindow -s TV;") -> (w1467:string)
                n877 = call "Param_Analysis_7_24b_JW.vi"("Independant Variable"=w1472, "error in (no error)"=w1480, "Data Folder"=w1482, "Parameter String"="Mobility-Sat (cm^2/Vs):", "Parameter Name"="Mobility-Sat", "Stats Folder"=w1481) -> ("error out"=w1475:errorcluster, "Output Array"=w1473:string[][], "Variables"=w1471:T27)  [unwired: 2 in, 1 out]
                n878 = call "Origin_Export_7_27a_JW.vi"("Input Conditions"=w1471, "Analysis Array"=w1473, "error in (no error)"=w1475, "Parameter Worksheet Name"="[MOBSTable]Mobilities", "Parameter Folder Script"="pe_cd \"Mobility-Sat\";", "Origin.IOApplication"=w1479) -> ("error out"=w1474:errorcluster, "reference out"=w1476:refnum<k7>)  [unwired: 3 in, 1 out]
                n879 = call "OAExecute.vi"("script"=w1467, "Error IO"=w1474, "Origin.IOApplication"=w1476) -> ()  [unwired: 1 in, 3 out]
              }
              frame #2 {
                n880 = local read "X Axis Display Type"() -> (w1485:string)
                n881 = local read "Opj X Axis"() -> (w1490:string)
                n882 = Concatenate Strings("window -a NSTSGraph;\nlayer.x.type=", w1490, "; layer.x.label.numFormat = ", w1485, "; Y3 = 1; X3 = 1;", "window -a NSTSTable;\nwindow -s TV;") -> (w1488:string)
                n883 = call "Param_Analysis_7_24b_JW.vi"("Independant Variable"=w1493, "error in (no error)"=w1496, "Data Folder"=w1494, "Parameter String"="Trap Density-STS (Traps/Vcm^2):", "Parameter Name"="Trap Density-STS", "Stats Folder"=w1495) -> ("error out"=w1500:errorcluster, "Output Array"=w1498:string[][], "Variables"=w1492:T27)  [unwired: 2 in, 1 out]
                n884 = call "Origin_Export_7_27a_JW.vi"("Input Conditions"=w1492, "Analysis Array"=w1498, "error in (no error)"=w1500, "Parameter Worksheet Name"="[NSTSTable]Trap Densities", "Parameter Folder Script"="pe_cd \"N-STS\";", "Origin.IOApplication"=w1497) -> ("error out"=w1499:errorcluster, "reference out"=w1501:refnum<k7>)  [unwired: 3 in, 1 out]
                n885 = call "OAExecute.vi"("script"=w1488, "Error IO"=w1499, "Origin.IOApplication"=w1501) -> ()  [unwired: 1 in, 3 out]
              }
              frame #3 {
                n886 = local read "X Axis Display Type"() -> (w1506:string)
                n887 = local read "Opj X Axis"() -> (w1511:string)
                n888 = call "Param_Analysis_7_24b_JW.vi"("Independant Variable"=w1514, "error in (no error)"=w1517, "Data Folder"=w1516, "Parameter String"="Trap Density-VT (Traps/Vcm^2):", "Parameter Name"="Trap Density-Vt", "Stats Folder"=w1515) -> ("error out"=w1521:errorcluster, "Output Array"=w1519:string[][], "Variables"=w1513:T27)  [unwired: 2 in, 1 out]
                n889 = Concatenate Strings("window -a NVtGraph;\nlayer.x.type=", w1511, "; layer.x.label.numFormat = ", w1506, "; Y3 = 1; X3 = 1;", "window -a NVtTable;\nwindow -s TV;") -> (w1509:string)
                n890 = call "Origin_Export_7_27a_JW.vi"("Input Conditions"=w1513, "Analysis Array"=w1519, "error in (no error)"=w1521, "Parameter Worksheet Name"="[NVTTable]Trap Densities", "Parameter Folder Script"="pe_cd \"N-Vt\";", "Origin.IOApplication"=w1518) -> ("error out"=w1520:errorcluster, "reference out"=w1522:refnum<k7>)  [unwired: 3 in, 1 out]
                n891 = call "OAExecute.vi"("script"=w1509, "Error IO"=w1520, "Origin.IOApplication"=w1522) -> ()  [unwired: 1 in, 3 out]
              }
              frame #4 {
                n892 = local read "X Axis Display Type"() -> (w1527:string)
                n893 = local read "Opj X Axis"() -> (w1532:string)
                n894 = Concatenate Strings("window -a OffIGraph;\nlayer.x.type=", w1532, "; layer.x.label.numFormat = ", w1527, "; Y3 = 1; X3 = 1;", "window -a OffITable;\nwindow -s TV;") -> (w1530:string)
                n895 = call "Param_Analysis_7_24b_JW.vi"("Independant Variable"=w1535, "error in (no error)"=w1538, "Data Folder"=w1536, "Parameter String"="Off I-Sat (A):", "Parameter Name"="Off I-Sat", "Stats Folder"=w1537) -> ("error out"=w1542:errorcluster, "Output Array"=w1540:string[][], "Variables"=w1534:T27)  [unwired: 2 in, 1 out]
                n896 = call "Origin_Export_7_27a_JW.vi"("Input Conditions"=w1534, "Analysis Array"=w1540, "error in (no error)"=w1542, "Parameter Worksheet Name"="[OffItable]OffCurrents", "Parameter Folder Script"="pe_cd \"OffI-Sat\";", "Origin.IOApplication"=w1539) -> ("error out"=w1541:errorcluster, "reference out"=w1543:refnum<k7>)  [unwired: 3 in, 1 out]
                n897 = call "OAExecute.vi"("script"=w1530, "Error IO"=w1541, "Origin.IOApplication"=w1543) -> ()  [unwired: 1 in, 3 out]
              }
              frame #5 {
                n898 = local read "X Axis Display Type"() -> (w1548:string)
                n899 = local read "Opj X Axis"() -> (w1553:string)
                n900 = Concatenate Strings("window -a OnOffGraph;\nlayer.x.type=", w1553, "; layer.x.label.numFormat = ", w1548, "; Y3 = 1; X3 = 1;", "window -a OnOffTable;\nwindow -s TV;") -> (w1551:string)
                n901 = call "Param_Analysis_7_24b_JW.vi"("Independant Variable"=w1556, "error in (no error)"=w1559, "Data Folder"=w1557, "Parameter String"="On/Off I-Sat:", "Parameter Name"="OnOff Ratio", "Stats Folder"=w1558) -> ("error out"=w1563:errorcluster, "Output Array"=w1561:string[][], "Variables"=w1555:T27)  [unwired: 2 in, 1 out]
                n902 = call "Origin_Export_7_27a_JW.vi"("Input Conditions"=w1555, "Analysis Array"=w1561, "error in (no error)"=w1563, "Parameter Worksheet Name"="[OnOffTable]On/Off Ratios", "Parameter Folder Script"="pe_cd \"OnOff-Ratio\";", "Origin.IOApplication"=w1560) -> ("error out"=w1562:errorcluster, "reference out"=w1564:refnum<k7>)  [unwired: 3 in, 1 out]
                n903 = call "OAExecute.vi"("script"=w1551, "Error IO"=w1562, "Origin.IOApplication"=w1564) -> ()  [unwired: 1 in, 3 out]
              }
              frame #6 {
                n904 = local read "X Axis Display Type"() -> (w1569:string)
                n905 = local read "Opj X Axis"() -> (w1574:string)
                n906 = call "Param_Analysis_7_24b_JW.vi"("Independant Variable"=w1577, "error in (no error)"=w1580, "Data Folder"=w1578, "Parameter String"="STS-Sat (V/decade):", "Parameter Name"="STS-Sat", "Stats Folder"=w1579) -> ("error out"=w1584:errorcluster, "Output Array"=w1582:string[][], "Variables"=w1576:T27)  [unwired: 2 in, 1 out]
                n907 = Concatenate Strings("window -a SGraph;\nlayer.x.type=", w1574, "; layer.x.label.numFormat = ", w1569, "; Y3 = 1; X3 = 1;", "window -a STable;\nwindow -s TV;") -> (w1572:string)
                n908 = call "Origin_Export_7_27a_JW.vi"("Input Conditions"=w1576, "Analysis Array"=w1582, "error in (no error)"=w1584, "Parameter Worksheet Name"="[STable]Threshold Swing", "Parameter Folder Script"="pe_cd \"STS-Sat\";", "Origin.IOApplication"=w1581) -> ("error out"=w1583:errorcluster, "reference out"=w1585:refnum<k7>)  [unwired: 3 in, 1 out]
                n909 = call "OAExecute.vi"("script"=w1572, "Error IO"=w1583, "Origin.IOApplication"=w1585) -> ()  [unwired: 1 in, 3 out]
              }
              frame #7 {
                n910 = local read "X Axis Display Type"() -> (w1590:string)
                n911 = local read "Opj X Axis"() -> (w1595:string)
                n912 = Concatenate Strings("window -a VtGraph;\nlayer.x.type=", w1595, "; layer.x.label.numFormat = ", w1590, "; Y3 = 1; X3 = 1;", "window -a VtTable;\nwindow -s TV;") -> (w1593:string)
                n913 = call "Param_Analysis_7_24b_JW.vi"("Independant Variable"=w1598, "error in (no error)"=w1603, "Data Folder"=w1601, "Parameter String"="Vt-Sat (V):", "Parameter Name"="Vt-Sat", "Stats Folder"=w1602) -> ("error out"=w1607:errorcluster, "Output Array"=w1605:string[][], "Variables"=w1597:T27)  [unwired: 2 in, 1 out]
                n914 = call "Origin_Export_7_27a_JW.vi"("Input Conditions"=w1597, "Analysis Array"=w1605, "error in (no error)"=w1607, "Parameter Worksheet Name"="[VtTable]Threshold Voltages", "Parameter Folder Script"="pe_cd \"Vt-Sat\";", "Origin.IOApplication"=w1604) -> ("error out"=w1606:errorcluster, "reference out"=w1608:refnum<k7>)  [unwired: 3 in, 1 out]
                n915 = call "OAExecute.vi"("script"=w1593, "Error IO"=w1606, "Origin.IOApplication"=w1608) -> ("Error IO Out"=w1599:errorcluster, "Origin.IOApplication"=w1600:refnum<k7>)  [unwired: 1 in, 1 out]
              }
            }
            n916 = Path To String(path=w1429) -> (string=w1428:string)
            n917 = call "OAExecute.vi"("script"="pe_cd /; ", "Error IO"=w1424, "Origin.IOApplication"=w1423) -> ("Error IO Out"=w1430:errorcluster, "Origin.IOApplication"=w1431:refnum<k7>)  [unwired: 1 in, 1 out]
            n918 = call <userlib>:"OASaveProject.vi"("path"=w1428, "Error IO"=w1430, "Origin.IOApplication"=w1431) -> ("Origin.IOApplication"=w1420:refnum<k7>)  [unwired: 2 out]
            n919 = call <userlib>:"OAEndSession.vi"("Origin.IOApplication"=w1420) -> ()  [unwired: 1 in, 3 out]
          }
        }
      }
    }
    "Current State" <- w11
    "Folder Index" <- w21
    n920 = Wait (ms)(milliseconds to wait=u32 50) -> ()  [unwired: 1 out]
    n921 = Equal?(x=w11, y=MegaAwesome_States."Exit") -> (x = y?=w14:bool)
  }
  n922 = disable-structure shown="Disabled" {
    disable-tunnel: w1 -> [w1617 _]
    frame Disabled {
      n923 = call "Close LabView?"("Enable"=w1617) -> ("OK"=w1616:bool)  [unwired: 17 in, 1 out]
      n924 = Quit LabVIEW(quit? (T)=w1616) -> ()
    }
    frame Enabled {
    }
  }
